vi "2D scan.vi"(5 "FIB Para":T4={"Z-step (nm)"=5.0, "Emission max"=4.0, "Emission min"=1.6, "Milling current (nA)"=1.2, "Enable alarm"=TRUE} {"Milling current (nA)" format="%.1g"}, 6 "Options":T6={"GetInfo"=TRUE, "Set Det A para"=TRUE, "Set WD"=FALSE, "Set Mag"=TRUE, "Set stig"=FALSE, "Display"=TRUE, "Save"=TRUE, "Detector A"=TRUE, "Detector B"=TRUE, "Detector C"=FALSE, "Detector D"=FALSE, "Inverse A"=FALSE, "Inverse B"=FALSE, "Inverse C"=FALSE, "Inverse D"=FALSE, "Inverse PNG"=FALSE, "Freeze"=TRUE, "PNG only"=TRUE}, 7 "File Info":cluster{"File path":path, "Notes":string}={"File path"=path "T:/Images", "Notes"=""}, 8 "Scan Para":T7={"X resolution"=1024, "Y resolution"=1024, "X center"=0.0, "Y center"=0.0, "X size (V)"=20.0, "Y size (V)"=20.0, "X stig"=0.0, "Y stig"=0.0, "Scan rate (Hz)"=1000000, "Oversampling"=4, "Read AI delay (samples)"=1, "Frame line rampdown ratio"=0.1, "Pixel size (nm)"=5.0, "WD"=4.0} {"WD" format="%#_7g"; "Frame line rampdown ratio" min=-1.0 max=1.0 step=0.05 format="%.2g"; "Scan rate (Hz)" max=4000000 format="%.2e"}, 9 "Det Info":T8={"Brightness A"=40.0, "Contrast A"=26.0, "Detector B name"="ESB @ 1.0 kV", "Brightness B"=40.0, "Contrast B"=40.0, "Detector C name"="PMT @ 6.0", "Detector D name"="Detector D"}, 10 "HW Config":T9={"SEM X coil"="PXI1Slot7/ao0", "SEM Y coil"="PXI1Slot7/ao1", "Detector A"="PXI1Slot7/ai0", "Detector B"="PXI1Slot7/ai1", "Detector C"="PXI1Slot7/ai2", "Detector D"="PXI1Slot7/ai3", "Det min (V)"=-10.0, "Det max (V)"=10.0, "COM port"="COM1", "Detector FIB-NI auto switch"="PXI1Slot7/port0/line0", "Machine Type"=0} {"Machine Type" items=["Feiss", "NVision"]}) -> (0 "Image Focus Index":T1, 1 "FIB parameters":T3, 2 "SEM parameters":T2={"Detector A"="", "Detector B"="Detecter B name", "Brightness A"=0.0, "Contrast A"=0.0, "Brightness B"=0.0, "Contrast B"=0.0, "Magnification"=0.0, "Pixel size"=0.0, "Working distance"=0.0, "EHT"=0.0, "Aperture"=0, "High current mode"=0, "Probe current"=0.0, "Scan rotation"=0.0, "Chamber vac"=0.0, "Gun vac"=0.0, "Beam shift X"=0.0, "Beam shift Y"=0.0, "Stig X"=0.0, "Stig Y"=0.0, "Alignment X"=0.0, "Alignment Y"=0.0, "Stage X"=0.0, "Stage Y"=0.0, "Stage Z"=0.0, "Stage T"=0.0, "Stage R"=0.0, "Stage M"=0.0}, 3 "Info & Status":T5={"AO SampClk.MaxRate"=2500000.0, "AI SampClk.MaxRate"=4000000.0, "AO rate"=1000000.0, "Scan speed"=4, "Detector number"=2, "X min (V)"=-10.0, "X max (V)"=10.0, "X min index"=0, "X max index"=1024, "AO multiline"=512, "Decimating factor"=2, "AvailSampPerChan"=17560, "AO scan line"=1024, "Total pixels recorded"=1048576, "Total lines scanned"=1024, "Scan time (m)"=0.0, "Scan time (s)"=1.153024, "Remaining time (m)"=0, "Remaining time (s)"=0} {"AvailSampPerChan" scale=0.0..1000000.0; "Scan time (s)" format="%.3f"; "Total pixels recorded" scale=0.0..1048576.0; "Scan speed" scale=1.0..15.0; "AO rate" format="%#_3e"})   [LabVIEW 2012]
uses:
  <vilib>/Utility/error.llb/DialogType.ctl
  <vilib>/DAQmx/write.llb/DAQmx Write (Digital Bool 1Line 1Point).vi
  <vilib>/DAQmx/read.llb/DAQmx Read (Raw 1D I16).vi
  <vilib>/DAQmx/write.llb/DAQmx Write (Analog 2D DBL NChan NSamp).vi
  <vilib>/DAQmx/create/channels.llb/DAQmx Create Channel (AI-Voltage-Basic).vi
  <vilib>/DAQmx/create/channels.llb/DAQmx Create Channel (AO-Voltage-Basic).vi
  <vilib>/DAQmx/create/channels.llb/DAQmx Create Channel (DO-Digital Output).vi
  <vilib>/DAQmx/miscellaneous.llb/DAQmx Fill In Error Info.vi
  <vilib>/DAQmx/configure/timing.llb/DAQmx Timing (Sample Clock).vi
  <vilib>/DAQmx/configure/trigger.llb/DAQmx Start Trigger (Digital Edge).vi
  <vilib>/Analysis/2dsp.llb/Decimate (single shot, DBL).vi
  <resource>/objmgr/daqmx.rc
  <vilib>/Analysis/NI_AALPro.lvlib
panel:
  out "PNG only":bool
  out "Eval D":i16[][](graph)
  out "Eval C":i16[][](graph)
  out "Eval B":i16[][](graph)
  out "Eval A":i16[][](graph)
  out "Freeze":bool
  out "Detector FIB-NI auto switch":tag
  out "GetInfo":bool
  out "Set X stig":bool=TRUE
  out "Y stig":dbl
  out "X stig":dbl
  out "Total time":dbl=1.153024
  in  "stop":bool=TRUE
  out "Det max (V)":dbl=10.0
  out "Det min (V)":dbl=-10.0
  out "Y max set":dbl=10.0
  out "Y min set":dbl=-10.0
  out "X max set":dbl=10.0
  out "X min set":dbl=-10.0
  in  "AvailSampPerChan":u32(slide)=17560 scale=0.0..1000000.0
  in  "AO scan line":u32=1024
  in  "AO multiline":u32=512
  in  "Decimating factor":u16=2
  in  "Remaining time (m)":u16
  in  "Remaining time (s)":u8
  in  "Scan time (s)":dbl=1.153024 format="%.3f"
  in  "Scan time (m)":dbl
  in  "Total lines scanned":i32=1024
  in  "Total pixels recorded":i32(slide)=1048576 scale=-1.0..1048576.0
  in  "X max (V)":dbl=10.0
  in  "X min (V)":dbl=-10.0
  in  "X min index":i32
  in  "X max index":i32=1024
  in  "Scan speed":u8(slide)=4 scale=1.0..15.0
  in  "AO rate":dbl=1000000.0 caption="Scanning rate" format="%#_3e"
  in  "Detector number":u8=2
  in  "AI SampClk.MaxRate":dbl=4000000.0
  in  "AO SampClk.MaxRate":dbl=2500000.0
  out "Det A Img":i16[][](graph)
  out "Det B Img":i16[][](graph)
  out "Det C Img":i16[][](graph)
  out "Det D Img":i16[][](graph)
  out "Notes":string
  out "File path":path=path "T:/Images/SW Tests"
  out "Inverse PNG":bool=TRUE
  out "Inverse D":bool
  out "Inverse C":bool
  out "Inverse B":bool
  out "Inverse A":bool
  out "Detector D":bool
  out "Detector C":bool
  out "Detector B":bool=TRUE
  out "Detector A":bool=TRUE
  out "Save":bool=TRUE
  out "Display":bool
  out "Set Mag":bool=TRUE
  out "Set WD":bool
  out "Set Det A para":bool=TRUE
  out "Z-step (nm)":dbl
  out "WD":dbl=6.0
  out "Pixel size (nm)":dbl=100.0
  out "Frame line rampdown ratio":dbl=0.1
  out "Read AI delay (samples)":i16=1
  out "Oversampling":u16=4
  out "Scan rate (Hz)":u32=1000000
  out "Y size (V)":dbl=20.0
  out "X size (V)":dbl=20.0
  out "Y center":dbl
  out "X center":dbl
  out "Y resolution":u32=1024
  out "X resolution":u32=1024
  out "Detector D name":string="Detector D"
  out "Detector C name":string="PMT @ 6.0"
  out "Contrast B":dbl=40.0
  out "Brightness B":dbl=40.0
  out "Detector B name":string="ESB @ 1.0 kV"
  out "Contrast A":dbl=26.0
  out "Brightness A":dbl=40.0
  out "COM port":refnum<visa-resource-name>="COM1"
  out "Det D I/O":tag="PXI1Slot3/ai3"
  out "Det C I/O":tag="PXI1Slot3/ai2"
  out "Det B I/O":tag="PXI1Slot3/ai1"
  out "Det A I/O":tag="PXI1Slot3/ai0"
  out "SEM Y coil":tag="PXI1Slot3/ao1"
  out "SEM X coil":tag="PXI1Slot3/ao0"
  out "File name":path=path "T:/Images/SW Tests/Y2010/M03/D26/Neon_10-03-26_153931.dat"
  out "Header done?":bool=TRUE
  # "Hardware Configuration"
  # "FIBBing Parameters"
  # "Detectors Information"
  # "Scanning Parameters"
  # "Emssion Alarm (uA)"
  # "Hz"
  # "Scanning time"
  # "m"
  # "s"
  # "Remaining time"
  # "m"
  # "s"
  # "Det"
  # "Detector A"
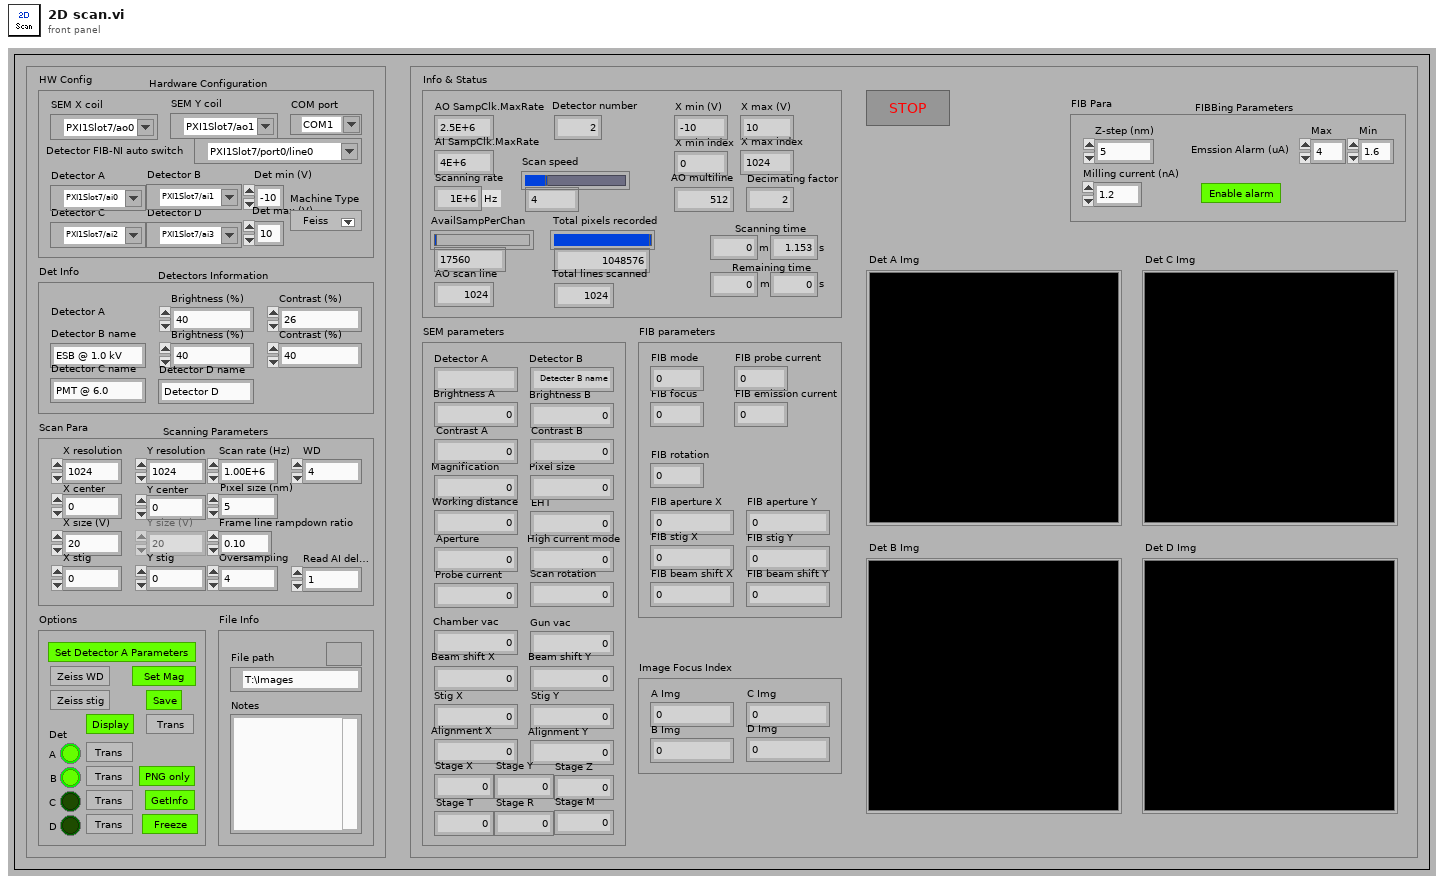
[diagram p1: front panel]
types:
  T1 = cluster{"A Img Focus Index":dbl, "B Img Focus Index":dbl, "C Img Focus Index":dbl, "D Img Focus Index":dbl}
  T2 = cluster{"Detector A":string, "Detector B":string, "Brightness A":sgl, "Contrast A":sgl, "Brightness B":sgl, "Contrast B":sgl, "Magnification":sgl, "Pixel size":sgl, "Working distance":sgl, "EHT":sgl, "Aperture":u8, "High current mode":u8, "Probe current":sgl, "Scan rotation":sgl, "Chamber vac":sgl, "Gun vac":sgl, "Beam shift X":sgl, "Beam shift Y":sgl, "Stig X":sgl, "Stig Y":sgl, "Alignment X":sgl, "Alignment Y":sgl, "Stage X":sgl, "Stage Y":sgl, "Stage Z":sgl, "Stage T":sgl, "Stage R":sgl, "Stage M":sgl}
  T3 = cluster{"FIB mode":u8, "FIB focus":sgl, "FIB probe current":u8, "FIB emission current":sgl, "FIB rotation":sgl, "FIB aperture X":sgl, "FIB aperture Y":sgl, "FIB stig X":sgl, "FIB stig Y":sgl, "FIB beam shift X":sgl, "FIB beam shift Y":sgl}
  T4 = cluster{"Z-step (nm)":dbl, "Emission max":dbl, "Emission min":dbl, "Milling current (nA)":sgl, "Enable alarm":bool}
  T5 = cluster{"AO SampClk.MaxRate":dbl, "AI SampClk.MaxRate":dbl, "AO rate":dbl, "Scan speed":u8, "Detector number":u8, "X min (V)":dbl, "X max (V)":dbl, "X min index":i32, "X max index":i32, "AO multiline":u32, "Decimating factor":u16, "AvailSampPerChan":u32, "AO scan line":u32, "Total pixels recorded":i32, "Total lines scanned":i32, "Scan time (m)":dbl, "Scan time (s)":dbl, "Remaining time (m)":u16, "Remaining time (s)":u8}
  T6 = cluster{"GetInfo":bool, "Set Det A para":bool, "Set WD":bool, "Set Mag":bool, "Set stig":bool, "Display":bool, "Save":bool, "Detector A":bool, "Detector B":bool, "Detector C":bool, "Detector D":bool, "Inverse A":bool, "Inverse B":bool, "Inverse C":bool, "Inverse D":bool, "Inverse PNG":bool, "Freeze":bool, "PNG only":bool}
  T7 = cluster{"X resolution":u32, "Y resolution":u32, "X center":dbl, "Y center":dbl, "X size (V)":dbl, "Y size (V)":dbl, "X stig":dbl, "Y stig":dbl, "Scan rate (Hz)":u32, "Oversampling":u16, "Read AI delay (samples)":i16, "Frame line rampdown ratio":dbl, "Pixel size (nm)":dbl, "WD":dbl}
  T8 = cluster{"Brightness A":dbl, "Contrast A":dbl, "Detector B name":string, "Brightness B":dbl, "Contrast B":dbl, "Detector C name":string, "Detector D name":string}
  T9 = cluster{"SEM X coil":tag, "SEM Y coil":tag, "Detector A":tag, "Detector B":tag, "Detector C":tag, "Detector D":tag, "Det min (V)":dbl, "Det max (V)":dbl, "COM port":refnum<visa-resource-name>, "Detector FIB-NI auto switch":tag, "Machine Type":u8}
  T10 = enum16{"SEM", "FIB", "Milling", "SEM + FIB", "Mill + SEM", "SEM Drift Correction", "FIB Drift Correction", "No Beam", "External", "External + SEM"}
  T11 = enum16{"open", "replace", "create", "open or create", "replace or create", "replace or create with confirmation"}
  T12 = typedef "DialogType.ctl" = u16
  T13 = cluster{"X resolution":u32, "Y resolution":u32, "Oversampling":u16, "Read AI delay (samples)":i16, "Scan speed":u8, "AO rate":dbl, "Frame line rampdown ratio":dbl, "X min (V)":dbl, "X max (V)":dbl}
  T14 = cluster{"Detector A":bool, "Detector B":bool, "Detector C":bool, "Detector D":bool}
  T15 = cluster{"Detector C name":string, "Detector D name":string}
  T16 = typedef "imagedata.ctl" = cluster{"image type":i32, "image depth":i32, "image":u8[], "mask":u8[], "colors":u32[], "Rectangle":cluster{"left":i16, "top":i16, "right":i16, "bottom":i16}}
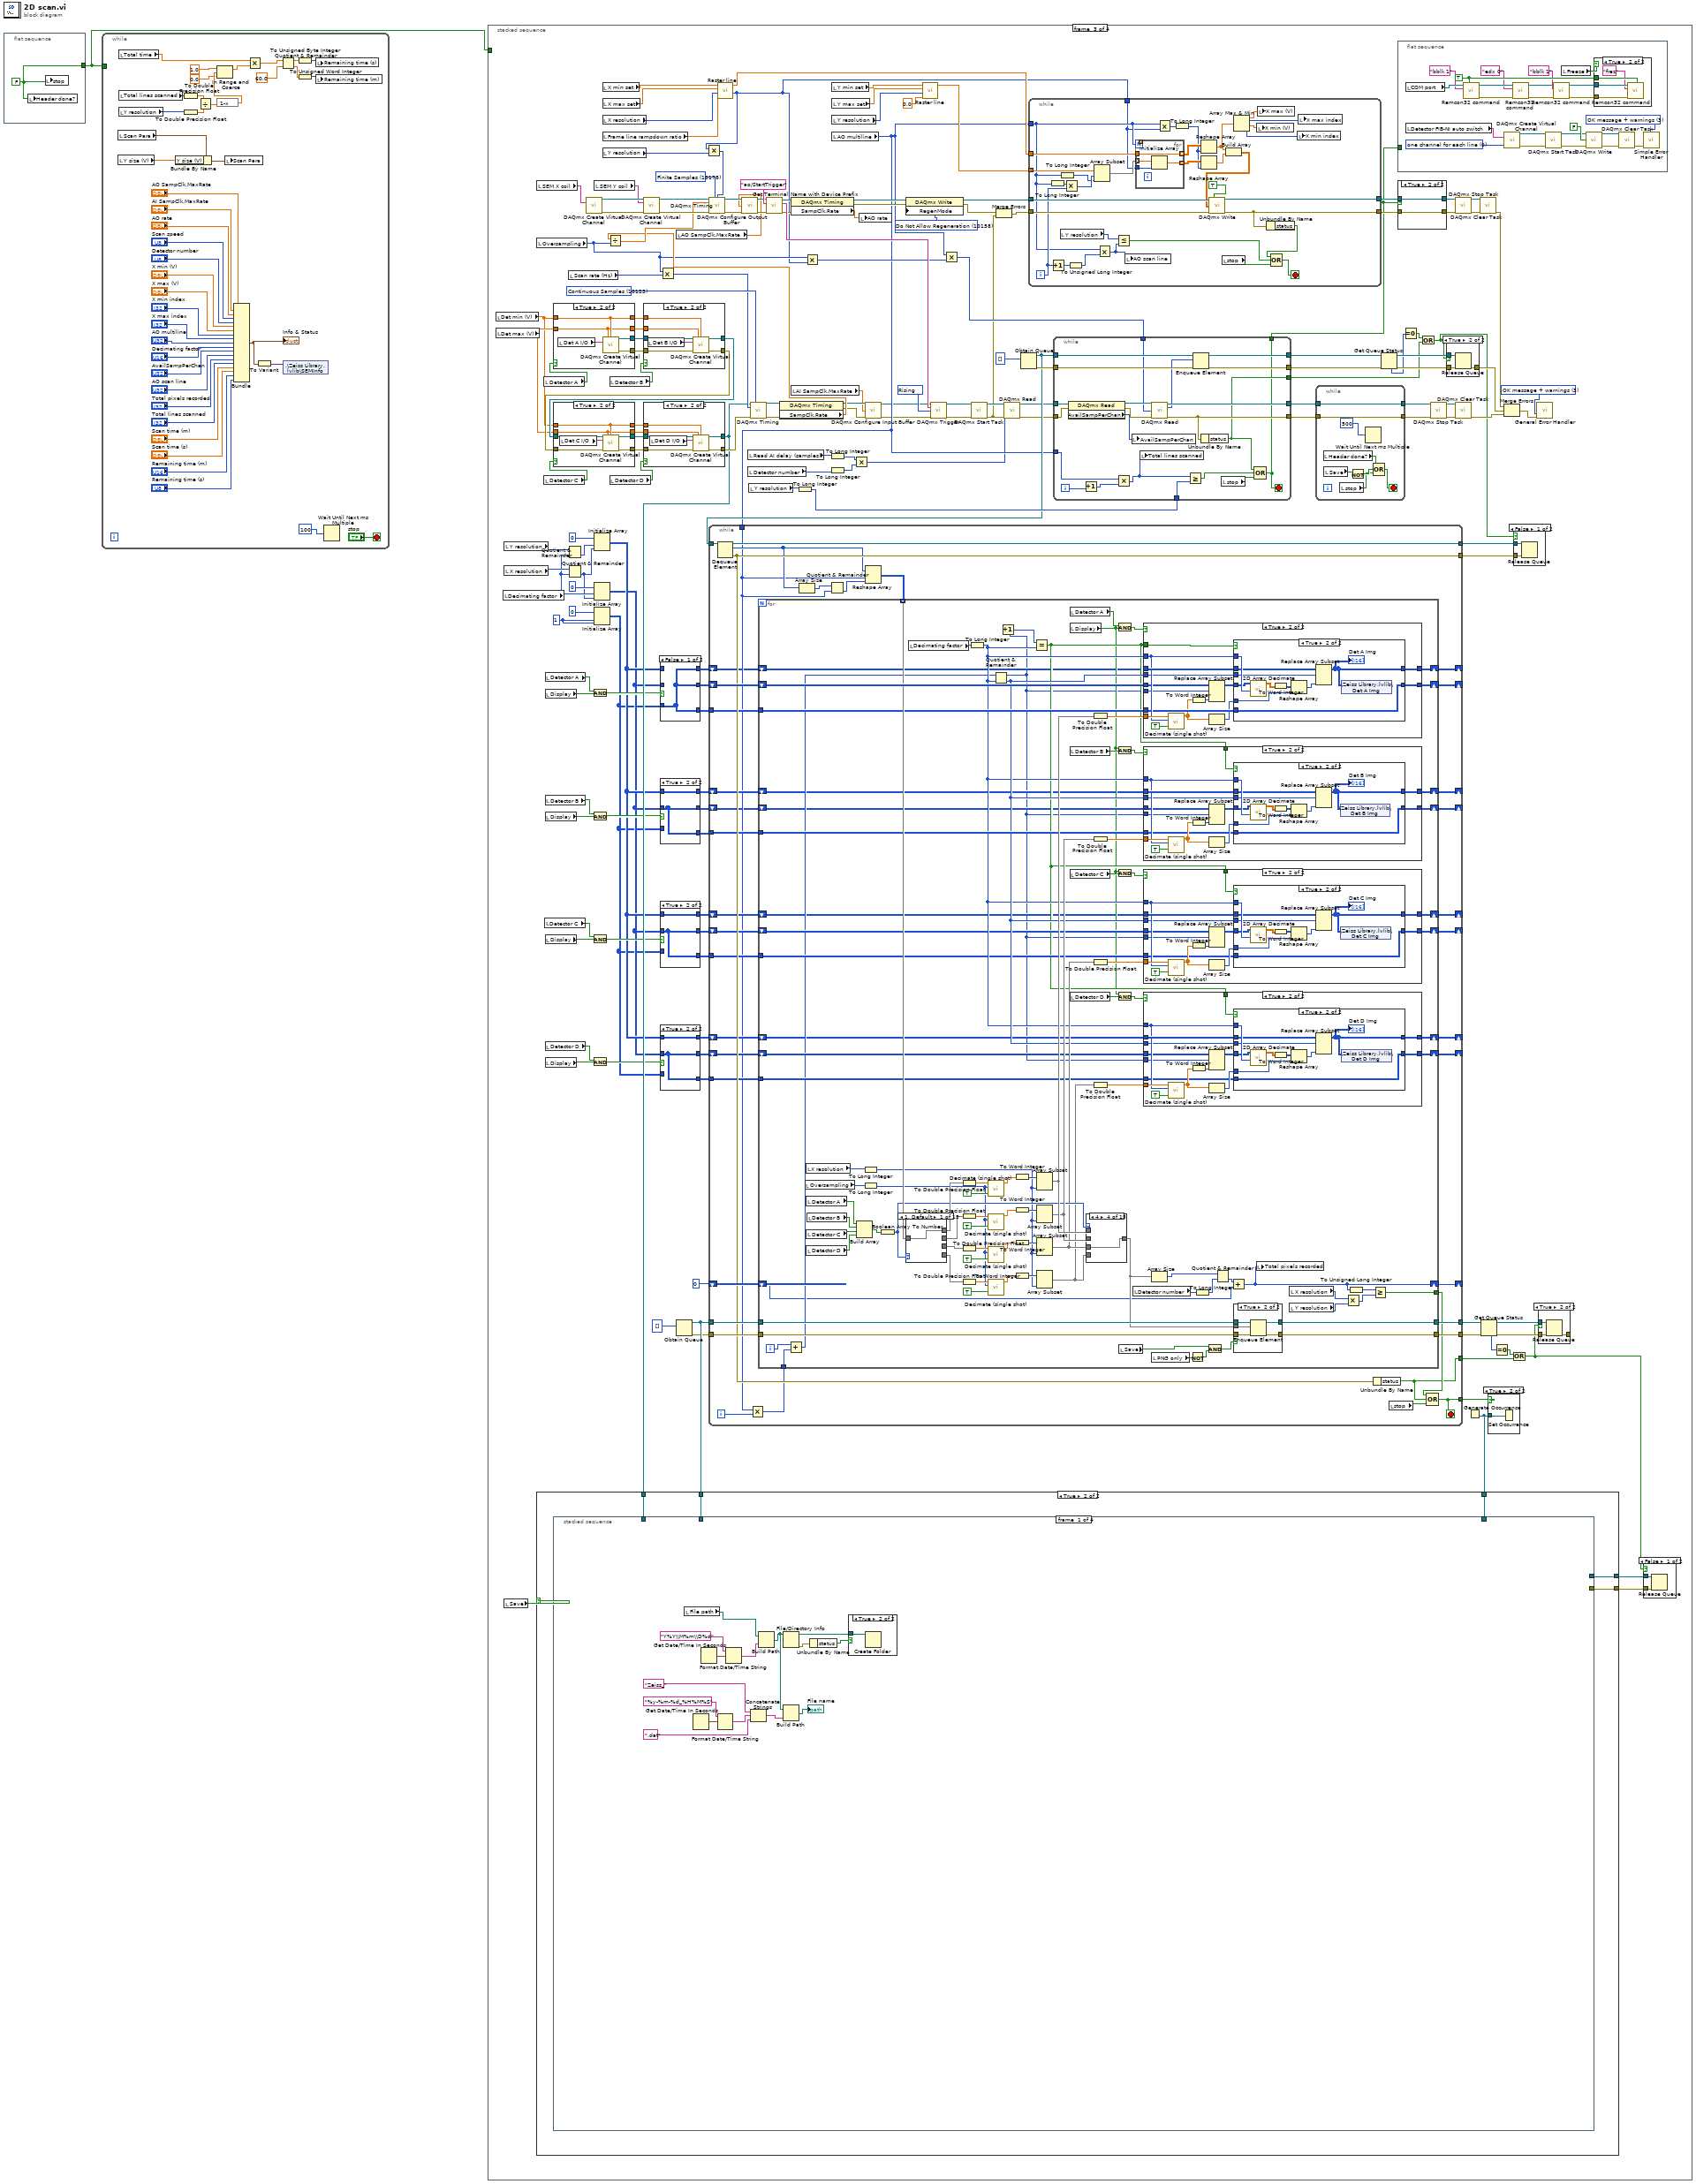
[diagram p0: block diagram]
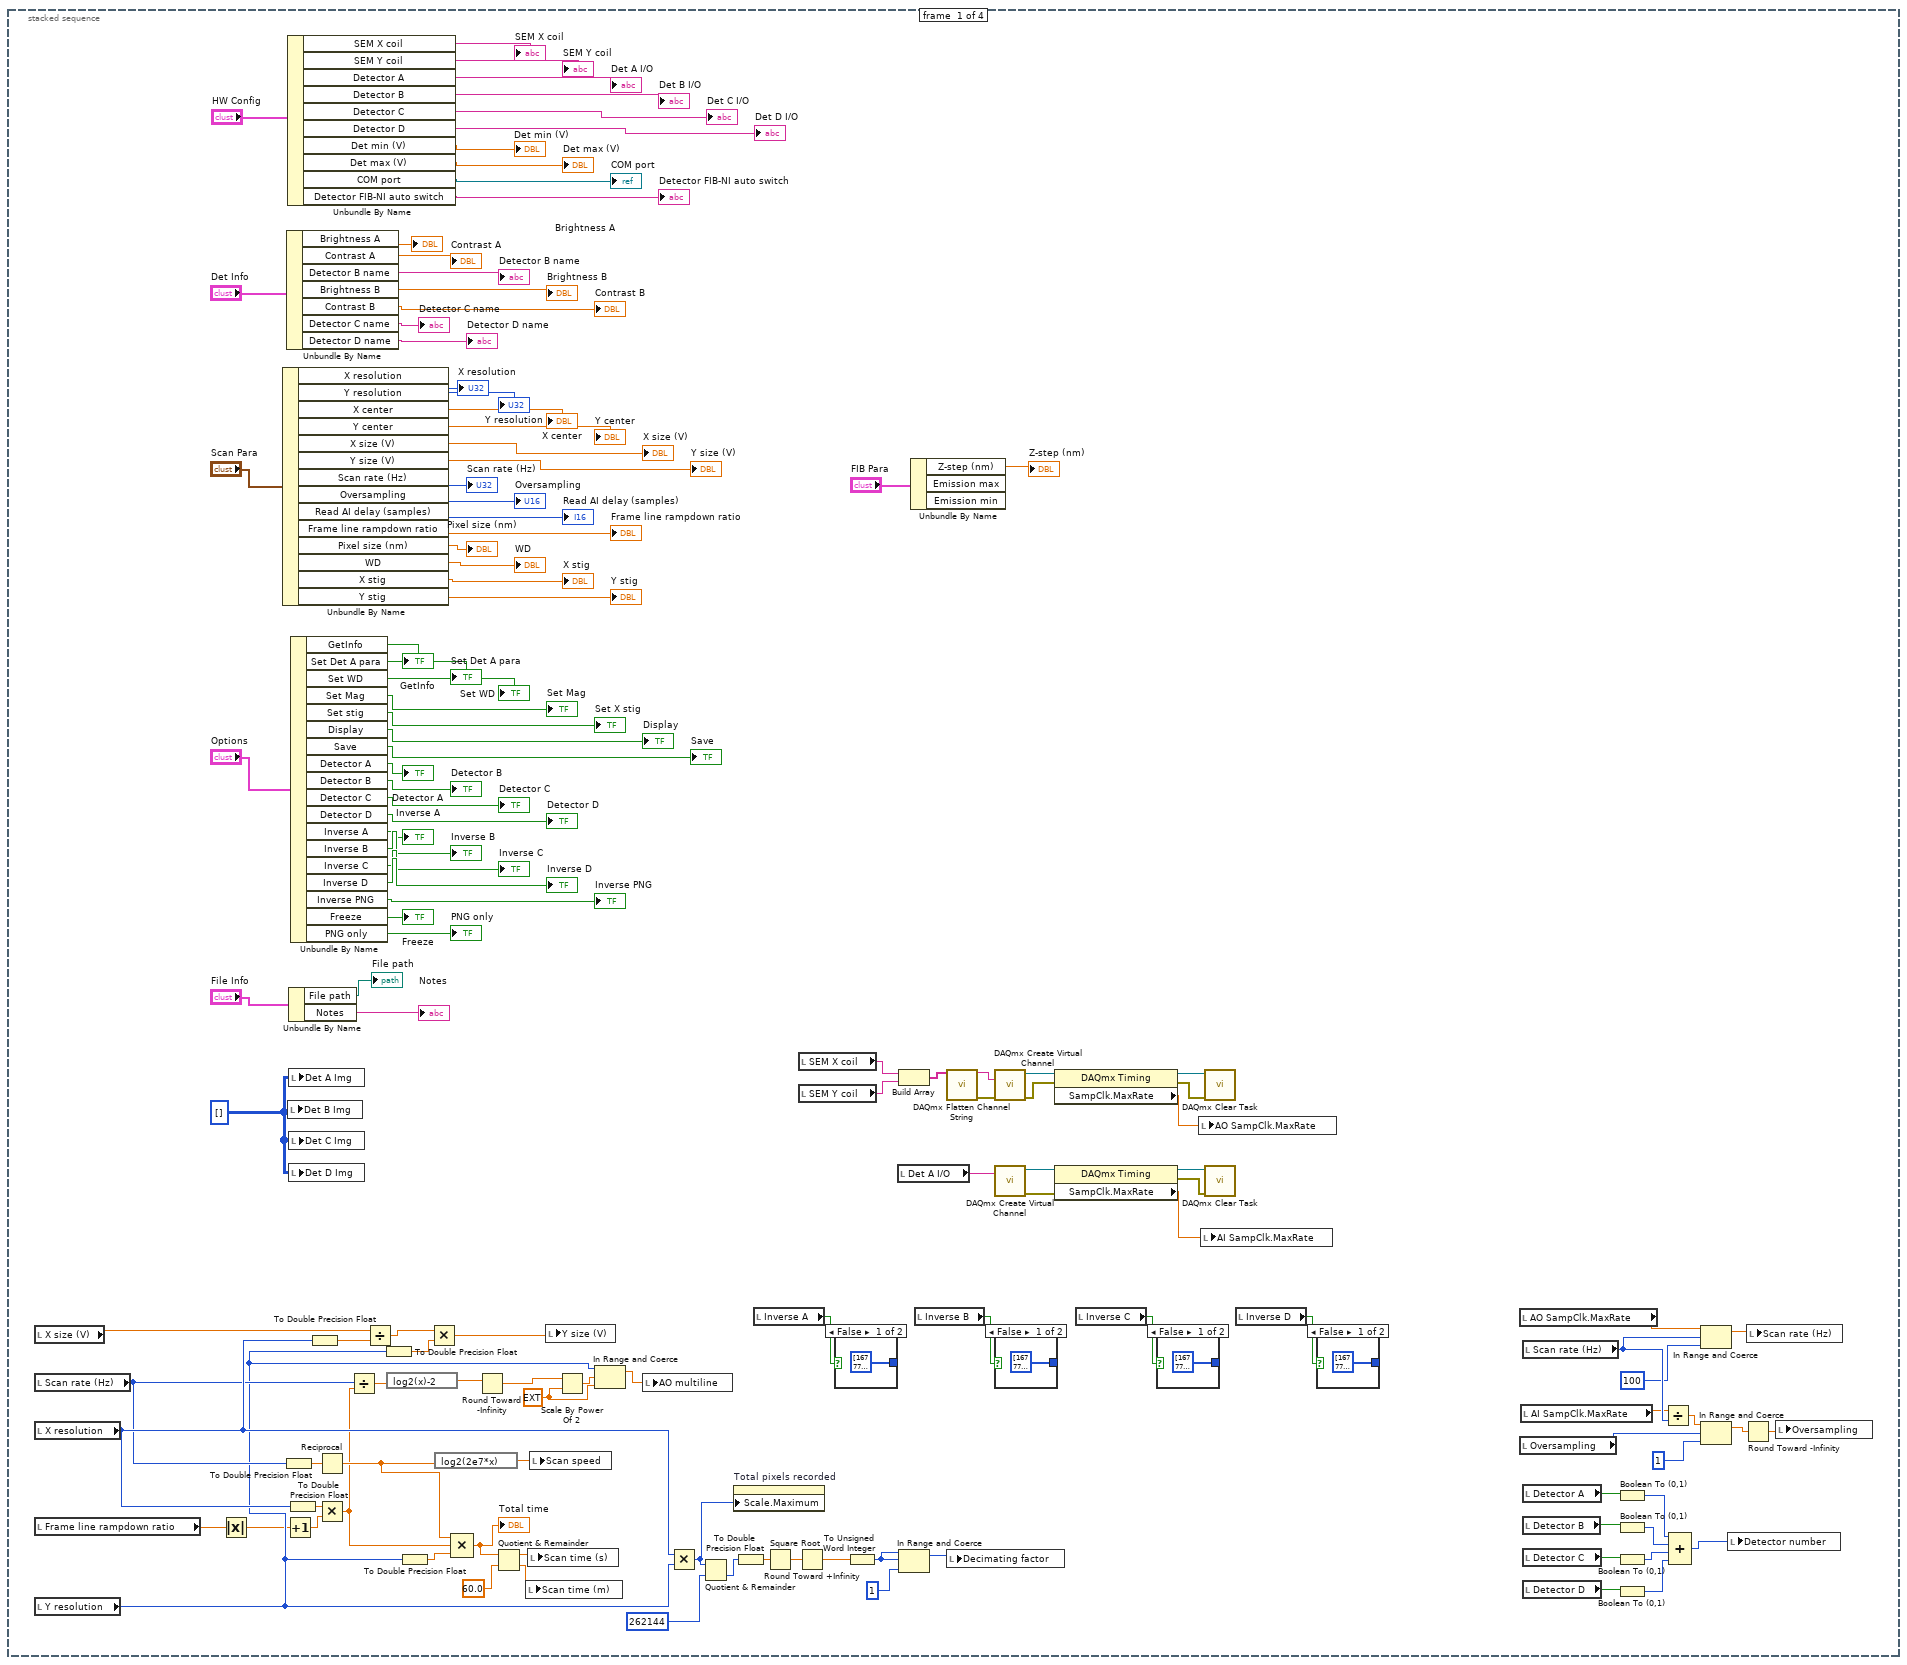
[diagram p2: hidden frame]
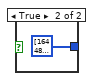
[diagram p3: hidden frame]
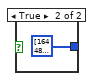
[diagram p4: hidden frame]
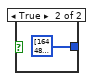
[diagram p5: hidden frame]
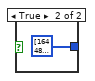
[diagram p6: hidden frame]
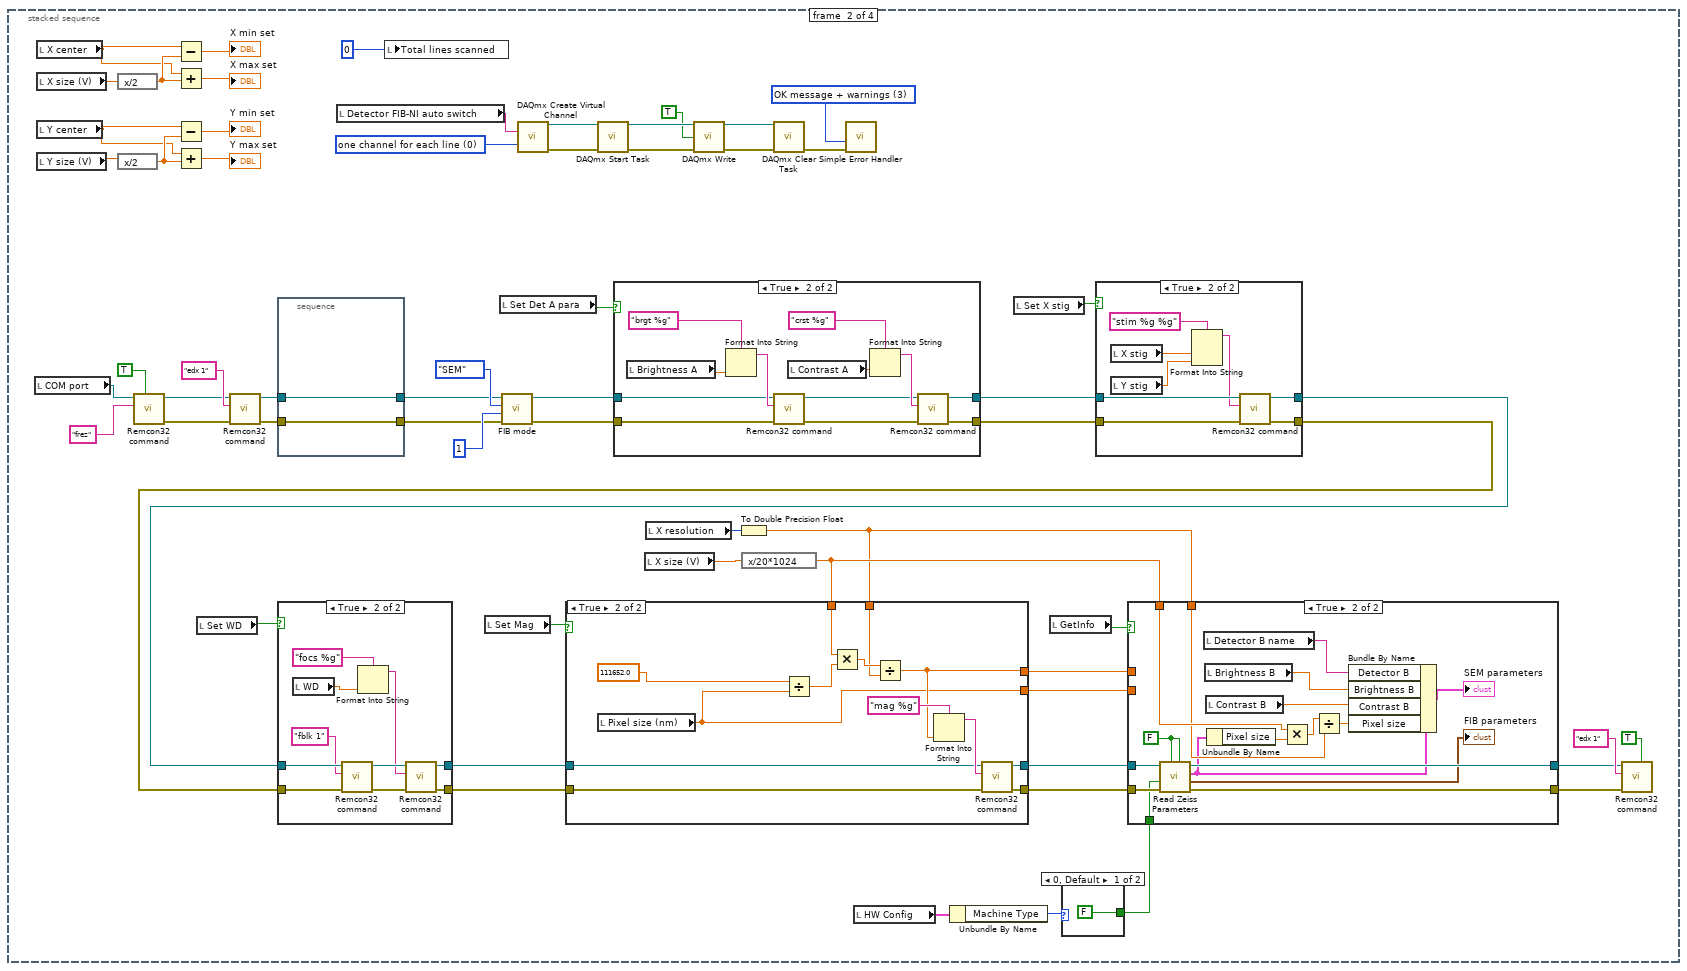
[diagram p7: hidden frame]
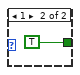
[diagram p8: hidden frame]
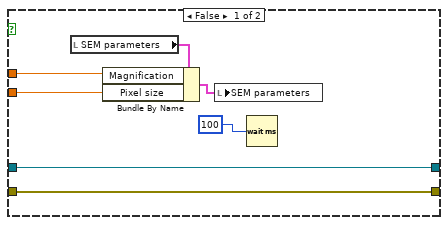
[diagram p9: hidden frame]
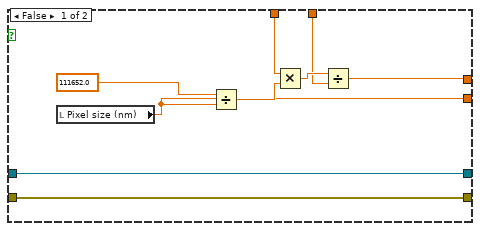
[diagram p12: hidden frame]
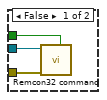
[diagram p14: hidden frame]
diagram:
  n1 = flat-sequence {
    tunnel: [w2] -> w1
    frame #0 {
      w2 = FALSE ("stop")
      n2 = local write "Header done?"(w2) -> ()
      n3 = local write "stop"(w2) -> ()
    }
  }
  n4 = while {
    tunnel: w1 -> [_]
    stop <- "stop" stop-if-true
    n5 = local read "Scan Para"() -> (w24:T7)
    n6 = local read "Y size (V)"() -> (w22:dbl)
    n7 = local read "Total time"() -> (w21:dbl)
    n8 = local read "Total lines scanned"() -> (w20:i32)
    n9 = local read "Y resolution"() -> (w9:u32)
    n10 = Bundle By Name(cluster=w24, "Y size (V)"=w22) -> (w23:T7)
    n11 = To Double Precision Float(number=w20) -> (double precision float=w13:dbl)
    n12 = To Double Precision Float(number=w9) -> (double precision float=w14:dbl)
    n13 = Divide(x=w13, y=w14) -> (x/y=w19:dbl)
    n14 = expression code="1-x"(w19) -> (w6:dbl)
    n15 = In Range and Coerce(upper limit=1.0, x=w6, lower limit=0.0) -> (coerced(x)=w3:dbl)  [unwired: 1 out]
    n16 = local write "Scan Para"(w23) -> ()
    n17 = Bundle("AO SampClk.MaxRate"="AO SampClk.MaxRate", "AI SampClk.MaxRate"="AI SampClk.MaxRate", "AO rate"="AO rate", "Scan speed"="Scan speed", "Detector number"="Detector number", "X min (V)"="X min (V)", "X max (V)"="X max (V)", "X min index"="X min index", "X max index"="X max index", "AO multiline"="AO multiline", "Decimating factor"="Decimating factor", "AvailSampPerChan"="AvailSampPerChan", "AO scan line"="AO scan line", "Total pixels recorded"="Total pixels recorded", "Total lines scanned"="Total lines scanned", "Scan time (m)"="Scan time (m)", "Scan time (s)"="Scan time (s)", "Remaining time (m)"="Remaining time (m)", "Remaining time (s)"="Remaining time (s)") -> (w7:T5)  [unwired: 1 out]
    "Info & Status" <- w7
    n18 = Multiply(x=w21, y=w3) -> (x*y=w15:dbl)
    n19 = To Variant(anything=w7) -> (Variant=w8:variant)
    n20 = Quotient & Remainder(x=w15, y=60.0) -> (x-y*floor(x/y)=w18:dbl, floor(x/y)=w17:dbl)
    n21 = shared-variable ".\\Zeiss Library.lvlib\\SEMInfo"(w8) -> ()  [unwired: 2 out]
    n22 = To Unsigned Byte Integer(number=w18) -> (unsigned 8bit integer=w11:u8)
    n23 = To Unsigned Word Integer(number=w17) -> (unsigned 16bit integer=w12:u16)
    n24 = local write "Remaining time (s)"(w11) -> ()
    n25 = local write "Remaining time (m)"(w12) -> ()
    n26 = Wait Until Next ms Multiple(millisecond multiple=u32 100) -> ()  [unwired: 1 out]
  }
  n27 = stacked-sequence {
    tunnel: w1 -> [_ _ _ _]
    frame #0 {
      w112 = i16[][] [] ("SEM")
      w164 = ext 1.0 ("x")
      n28 = local read "X size (V)"() -> (w167:dbl)
      n29 = local read "Scan rate (Hz)"() -> (w169:u32)
      n30 = local read "X resolution"() -> (w170:u32)
      n31 = local read "Frame line rampdown ratio"() -> (w171:dbl)
      n32 = local read "Y resolution"() -> (w168:u32)
      n33 = Absolute Value(x=w171) -> (abs(x)=w51:dbl)
      n34 = Unbundle By Name("Scan Para") -> ("X resolution"=→"X resolution":u32, "Y resolution"=→"Y resolution":u32, "X center"=→"X center":dbl, "Y center"=→"Y center":dbl, "X size (V)"=→"X size (V)":dbl, "Y size (V)"=→"Y size (V)":dbl, "Scan rate (Hz)"=→"Scan rate (Hz)":u32, "Oversampling"=→"Oversampling":u16, "Read AI delay (samples)"=→"Read AI delay (samples)":i16, "Frame line rampdown ratio"=→"Frame line rampdown ratio":dbl, "Pixel size (nm)"=→"Pixel size (nm)":dbl, "WD"=→"WD":dbl, "X stig"=→"X stig":dbl, "Y stig"=→"Y stig":dbl)
      n35 = To Double Precision Float(number=w169) -> (double precision float=w154:dbl)
      n36 = Increment(x=w51) -> (x+1=w149:dbl)
      n37 = Unbundle By Name("Det Info") -> ("Brightness A"=→"Brightness A":dbl, "Contrast A"=→"Contrast A":dbl, "Detector B name"=→"Detector B name":string, "Brightness B"=→"Brightness B":dbl, "Contrast B"=→"Contrast B":dbl, "Detector C name"=→"Detector C name":string, "Detector D name"=→"Detector D name":string)
      n38 = Unbundle By Name("HW Config") -> ("SEM X coil"=→"SEM X coil":tag, "SEM Y coil"=→"SEM Y coil":tag, "Detector A"=→"Det A I/O":tag, "Detector B"=→"Det B I/O":tag, "Detector C"=→"Det C I/O":tag, "Detector D"=→"Det D I/O":tag, "Det min (V)"=→"Det min (V)":dbl, "Det max (V)"=→"Det max (V)":dbl, "COM port"=→"COM port":refnum<visa-resource-name>, "Detector FIB-NI auto switch"=→"Detector FIB-NI auto switch":tag)
      n39 = local write "Det B Img"(w112) -> ()
      n40 = To Double Precision Float(number=w170) -> (double precision float=w155:dbl)
      n41 = Unbundle By Name("File Info") -> ("File path"=→"File path":path, "Notes"=→"Notes":string)
      n42 = local write "Det A Img"(w112) -> ()
      n43 = local write "Det C Img"(w112) -> ()
      n44 = local write "Det D Img"(w112) -> ()
      n45 = Unbundle By Name("Options") -> ("GetInfo"=→"GetInfo":bool, "Set Det A para"=→"Set Det A para":bool, "Set WD"=→"Set WD":bool, "Set Mag"=→"Set Mag":bool, "Set stig"=→"Set X stig":bool, "Display"=→"Display":bool, "Save"=→"Save":bool, "Detector A"=→"Detector A":bool, "Detector B"=→"Detector B":bool, "Detector C"=→"Detector C":bool, "Detector D"=→"Detector D":bool, "Inverse A"=→"Inverse A":bool, "Inverse B"=→"Inverse B":bool, "Inverse C"=→"Inverse C":bool, "Inverse D"=→"Inverse D":bool, "Inverse PNG"=→"Inverse PNG":bool, "Freeze"=→"Freeze":bool, "PNG only"=→"PNG only":bool)
      n46 = To Double Precision Float(number=w170) -> (double precision float=w153:dbl)
      n47 = Reciprocal(x=w154) -> (1/x=w150:dbl)
      n48 = Multiply(x=w155, y=w149) -> (x*y=w49:dbl)
      n49 = Divide(x=w169, y=w49) -> (x/y=w161:dbl)
      n50 = Divide(x=w167, y=w153) -> (x/y=w152:dbl)
      n51 = To Double Precision Float(number=w168) -> (double precision float=w156:dbl)
      n52 = expression code="log2(x)-2"(w161) -> (w162:dbl)
      n53 = To Double Precision Float(number=w168) -> (double precision float=w157:dbl)
      n54 = Multiply(x=w152, y=w156) -> (x*y=w166:dbl)
      n55 = expression code="log2(2e7*x)"(w150) -> (w172:dbl)
      n56 = Compound Arithmetic op=MULTIPLY(w150, w49, w157) -> (w151:dbl)
      "Total time" <- w151
      n57 = Round Toward -Infinity(1:w162) -> (0:w165:dbl)
      n58 = Quotient & Remainder(x=w151, y=60.0) -> (x-y*floor(x/y)=w174:dbl, floor(x/y)=w173:dbl)
      n59 = local write "Scan time (m)"(w173) -> ()
      n60 = local write "Scan time (s)"(w174) -> ()
      n61 = local write "Scan speed"(w172) -> ()
      n62 = local write "Y size (V)"(w166) -> ()
      n63 = Scale By Power Of 2(n=w165, x=w164) -> (x*2^n=w163:ext)
      n64 = In Range and Coerce(upper limit=w168, x=w163, lower limit=w164) -> (coerced(x)=w50:ext)  [unwired: 1 out]
      n65 = local write "AO multiline"(w50) -> ()
      n66 = Multiply(x=w170, y=w168) -> (x*y=w148:u32)
      n67 = Quotient & Remainder(x=w148, y=u32 262144) -> (floor(x/y)=w146:u32)  [unwired: 1 out]
      n68 = property on="Total pixels recorded" class="Slide (strict)"("Scale.Maximum"=w148) -> ()  [unwired: 2 in, 2 out]
      n69 = To Double Precision Float(number=w146) -> (double precision float=w159:dbl)
      n70 = local read "Inverse A"() -> (w175:bool)
      n71 = Square Root(x=w159) -> (sqrt(x)=w147:dbl)
      n72 = Round Toward +Infinity(x=w147) -> (ceil(x): smallest int >= x=w160:dbl)
      n73 = local read "SEM X coil"() -> (w115:tag)
      n74 = local read "SEM Y coil"() -> (w114:tag)
      n75 = case shown="False" w175 {
        tunnel: [u32[] [16777222, 65793, 131586, 197379, 263172, 328965, 394758, 460551, 526344, 592137, 657930, 723723, 789516, 855309, 921102, 986895, 1052688, 1118481, 1184274, 1250067, 1315860, 1381653, 1447446, 1513239, 1579032, 1644825, 1710618, 1776411, 1842204, 1907997, 1973790, 2039583, 2105376, 2171169, 2236962, 2302755, 2368548, 2434341, 2500134, 2565927, 2631720, 2697513, 2763306, 2829099, 2894892, 2960685, 3026478, 3092271, 3158064, 3223857, 3289650, 3355443, 3421236, 3487029, 3552822, 3618615, 3684408, 3750201, 3815994, 3881787, 3947580, 4013373, 4079166, 4144959, 4210752, 4276545, 4342338, 4408131, 4473924, 4539717, 4605510, 4671303, 4737096, 4802889, 4868682, 4934475, 5000268, 5066061, 5131854, 5197647, 5263440, 5329233, 5395026, 5460819, 5526612, 5592405, 5658198, 5723991, 5789784, 5855577, 5921370, 5987163, 6052956, 6118749, 6184542, 6250335, 6316128, 6381921, 6447714, 6513507, 6579300, 6645093, 6710886, 6776679, 6842472, 6908265, 6974058, 7039851, 7105644, 7171437, 7237230, 7303023, 7368816, 7434609, 7500402, 7566195, 7631988, 7697781, 7763574, 7829367, 7895160, 7960953, 8026746, 8092539, 8158332, 8224125, 8289918, 8355711, 8421504, 8487297, 8553090, 8618883, 8684676, 8750469, 8816262, 8882055, 8947848, 9013641, 9079434, 9145227, 9211020, 9276813, 9342606, 9408399, 9474192, 9539985, 9605778, 9671571, 9737364, 9803157, 9868950, 9934743, 10000536, 10066329, 10132122, 10197915, 10263708, 10329501, 10395294, 10461087, 10526880, 10592673, 10658466, 10724259, 10790052, 10855845, 10921638, 10987431, 11053224, 11119017, 11184810, 11250603, 11316396, 11382189, 11447982, 11513775, 11579568, 11645361, 11711154, 11776947, 11842740, 11908533, 11974326, 12040119, 12105912, 12171705, 12237498, 12303291, 12369084, 12434877, 12500670, 12566463, 12632256, 12698049, 12763842, 12829635, 12895428, 12961221, 13027014, 13092807, 13158600, 13224393, 13290186, 13355979, 13421772, 13487565, 13553358, 13619151, 13684944, 13750737, 13816530, 13882323, 13948116, 14013909, 14079702, 14145495, 14211288, 14277081, 14342874, 14408667, 14474460, 14540253, 14606046, 14671839, 14737632, 14803425, 14869218, 14935011, 15000804, 15066597, 15132390, 15198183, 15263976, 15329769, 15395562, 15461355, 15527148, 15592941, 15658734, 15724527, 15790320, 15856113, 15921906, 15987699, 16053492, 16119285, 16185078, 16250871, 16316664, 16382457, 16448250, 16514043, 16579836, 16645629, 16711422, 16448250] ("256 gray scale") u32[] [16448250, 16711422, 16645629, 16579836, 16514043, 16448250, 16382457, 16316664, 16250871, 16185078, 16119285, 16053492, 15987699, 15921906, 15856113, 15790320, 15724527, 15658734, 15592941, 15527148, 15461355, 15395562, 15329769, 15263976, 15198183, 15132390, 15066597, 15000804, 14935011, 14869218, 14803425, 14737632, 14671839, 14606046, 14540253, 14474460, 14408667, 14342874, 14277081, 14211288, 14145495, 14079702, 14013909, 13948116, 13882323, 13816530, 13750737, 13684944, 13619151, 13553358, 13487565, 13421772, 13355979, 13290186, 13224393, 13158600, 13092807, 13027014, 12961221, 12895428, 12829635, 12763842, 12698049, 12632256, 12566463, 12500670, 12434877, 12369084, 12303291, 12237498, 12171705, 12105912, 12040119, 11974326, 11908533, 11842740, 11776947, 11711154, 11645361, 11579568, 11513775, 11447982, 11382189, 11316396, 11250603, 11184810, 11119017, 11053224, 10987431, 10921638, 10855845, 10790052, 10724259, 10658466, 10592673, 10526880, 10461087, 10395294, 10329501, 10263708, 10197915, 10132122, 10066329, 10000536, 9934743, 9868950, 9803157, 9737364, 9671571, 9605778, 9539985, 9474192, 9408399, 9342606, 9276813, 9211020, 9145227, 9079434, 9013641, 8947848, 8882055, 8816262, 8750469, 8684676, 8618883, 8553090, 8487297, 8421504, 8355711, 8289918, 8224125, 8158332, 8092539, 8026746, 7960953, 7895160, 7829367, 7763574, 7697781, 7631988, 7566195, 7500402, 7434609, 7368816, 7303023, 7237230, 7171437, 7105644, 7039851, 6974058, 6908265, 6842472, 6776679, 6710886, 6645093, 6579300, 6513507, 6447714, 6381921, 6316128, 6250335, 6184542, 6118749, 6052956, 5987163, 5921370, 5855577, 5789784, 5723991, 5658198, 5592405, 5526612, 5460819, 5395026, 5329233, 5263440, 5197647, 5131854, 5066061, 5000268, 4934475, 4868682, 4802889, 4737096, 4671303, 4605510, 4539717, 4473924, 4408131, 4342338, 4276545, 4210752, 4144959, 4079166, 4013373, 3947580, 3881787, 3815994, 3750201, 3684408, 3618615, 3552822, 3487029, 3421236, 3355443, 3289650, 3223857, 3158064, 3092271, 3026478, 2960685, 2894892, 2829099, 2763306, 2697513, 2631720, 2565927, 2500134, 2434341, 2368548, 2302755, 2236962, 2171169, 2105376, 2039583, 1973790, 1907997, 1842204, 1776411, 1710618, 1644825, 1579032, 1513239, 1447446, 1381653, 1315860, 1250067, 1184274, 1118481, 1052688, 986895, 921102, 855309, 789516, 723723, 657930, 592137, 526344, 460551, 394758, 328965, 263172, 197379, 131586, 65793, 16777222] ("256 gray scale inverse")] -> _
        frame False {
        }
        frame True {
        }
      }
      n76 = To Unsigned Word Integer(number=w160) -> (unsigned 16bit integer=w48:u16)
      n77 = local read "Det A I/O"() -> (w121:tag)
      n78 = Build Array(w115, w114) -> (w113:tag[])
      n79 = In Range and Coerce(upper limit=w48, x=w48, lower limit=u16 1) -> (coerced(x)=w47:u16)  [unwired: 1 out]
      n80 = Unbundle By Name("FIB Para") -> ("Z-step (nm)"=→"Z-step (nm)":dbl)  [unwired: 2 out]
      n81 = local read "Inverse B"() -> (w176:bool)
      n82 = call <vilib>:"DAQmx Flatten Channel String.vi"("names in"=w113) -> ("names out"=w116:string, "error out"=w54:errorcluster)  [unwired: 1 in, 12 out]
      n83 = local write "Decimating factor"(w47) -> ()
      n84 = call-poly <vilib>:"DAQmx Create Virtual Channel.vi"("physical channels"=w116, "error in"=w54) -> ("task out"=w125:refnum<k21>, "error out"=w120:errorcluster)  [unwired: 7 in, 5 out]
      n85 = call-poly <vilib>:"DAQmx Create Virtual Channel.vi"("physical channels"=w121) -> ("task out"=w122:refnum<k21>, "error out"=w117:errorcluster)  [unwired: 8 in, 5 out]
      n86 = case shown="False" w176 {
        tunnel: [u32[] [16777222, 65793, 131586, 197379, 263172, 328965, 394758, 460551, 526344, 592137, 657930, 723723, 789516, 855309, 921102, 986895, 1052688, 1118481, 1184274, 1250067, 1315860, 1381653, 1447446, 1513239, 1579032, 1644825, 1710618, 1776411, 1842204, 1907997, 1973790, 2039583, 2105376, 2171169, 2236962, 2302755, 2368548, 2434341, 2500134, 2565927, 2631720, 2697513, 2763306, 2829099, 2894892, 2960685, 3026478, 3092271, 3158064, 3223857, 3289650, 3355443, 3421236, 3487029, 3552822, 3618615, 3684408, 3750201, 3815994, 3881787, 3947580, 4013373, 4079166, 4144959, 4210752, 4276545, 4342338, 4408131, 4473924, 4539717, 4605510, 4671303, 4737096, 4802889, 4868682, 4934475, 5000268, 5066061, 5131854, 5197647, 5263440, 5329233, 5395026, 5460819, 5526612, 5592405, 5658198, 5723991, 5789784, 5855577, 5921370, 5987163, 6052956, 6118749, 6184542, 6250335, 6316128, 6381921, 6447714, 6513507, 6579300, 6645093, 6710886, 6776679, 6842472, 6908265, 6974058, 7039851, 7105644, 7171437, 7237230, 7303023, 7368816, 7434609, 7500402, 7566195, 7631988, 7697781, 7763574, 7829367, 7895160, 7960953, 8026746, 8092539, 8158332, 8224125, 8289918, 8355711, 8421504, 8487297, 8553090, 8618883, 8684676, 8750469, 8816262, 8882055, 8947848, 9013641, 9079434, 9145227, 9211020, 9276813, 9342606, 9408399, 9474192, 9539985, 9605778, 9671571, 9737364, 9803157, 9868950, 9934743, 10000536, 10066329, 10132122, 10197915, 10263708, 10329501, 10395294, 10461087, 10526880, 10592673, 10658466, 10724259, 10790052, 10855845, 10921638, 10987431, 11053224, 11119017, 11184810, 11250603, 11316396, 11382189, 11447982, 11513775, 11579568, 11645361, 11711154, 11776947, 11842740, 11908533, 11974326, 12040119, 12105912, 12171705, 12237498, 12303291, 12369084, 12434877, 12500670, 12566463, 12632256, 12698049, 12763842, 12829635, 12895428, 12961221, 13027014, 13092807, 13158600, 13224393, 13290186, 13355979, 13421772, 13487565, 13553358, 13619151, 13684944, 13750737, 13816530, 13882323, 13948116, 14013909, 14079702, 14145495, 14211288, 14277081, 14342874, 14408667, 14474460, 14540253, 14606046, 14671839, 14737632, 14803425, 14869218, 14935011, 15000804, 15066597, 15132390, 15198183, 15263976, 15329769, 15395562, 15461355, 15527148, 15592941, 15658734, 15724527, 15790320, 15856113, 15921906, 15987699, 16053492, 16119285, 16185078, 16250871, 16316664, 16382457, 16448250, 16514043, 16579836, 16645629, 16711422, 16448250] ("256 gray scale") u32[] [16448250, 16711422, 16645629, 16579836, 16514043, 16448250, 16382457, 16316664, 16250871, 16185078, 16119285, 16053492, 15987699, 15921906, 15856113, 15790320, 15724527, 15658734, 15592941, 15527148, 15461355, 15395562, 15329769, 15263976, 15198183, 15132390, 15066597, 15000804, 14935011, 14869218, 14803425, 14737632, 14671839, 14606046, 14540253, 14474460, 14408667, 14342874, 14277081, 14211288, 14145495, 14079702, 14013909, 13948116, 13882323, 13816530, 13750737, 13684944, 13619151, 13553358, 13487565, 13421772, 13355979, 13290186, 13224393, 13158600, 13092807, 13027014, 12961221, 12895428, 12829635, 12763842, 12698049, 12632256, 12566463, 12500670, 12434877, 12369084, 12303291, 12237498, 12171705, 12105912, 12040119, 11974326, 11908533, 11842740, 11776947, 11711154, 11645361, 11579568, 11513775, 11447982, 11382189, 11316396, 11250603, 11184810, 11119017, 11053224, 10987431, 10921638, 10855845, 10790052, 10724259, 10658466, 10592673, 10526880, 10461087, 10395294, 10329501, 10263708, 10197915, 10132122, 10066329, 10000536, 9934743, 9868950, 9803157, 9737364, 9671571, 9605778, 9539985, 9474192, 9408399, 9342606, 9276813, 9211020, 9145227, 9079434, 9013641, 8947848, 8882055, 8816262, 8750469, 8684676, 8618883, 8553090, 8487297, 8421504, 8355711, 8289918, 8224125, 8158332, 8092539, 8026746, 7960953, 7895160, 7829367, 7763574, 7697781, 7631988, 7566195, 7500402, 7434609, 7368816, 7303023, 7237230, 7171437, 7105644, 7039851, 6974058, 6908265, 6842472, 6776679, 6710886, 6645093, 6579300, 6513507, 6447714, 6381921, 6316128, 6250335, 6184542, 6118749, 6052956, 5987163, 5921370, 5855577, 5789784, 5723991, 5658198, 5592405, 5526612, 5460819, 5395026, 5329233, 5263440, 5197647, 5131854, 5066061, 5000268, 4934475, 4868682, 4802889, 4737096, 4671303, 4605510, 4539717, 4473924, 4408131, 4342338, 4276545, 4210752, 4144959, 4079166, 4013373, 3947580, 3881787, 3815994, 3750201, 3684408, 3618615, 3552822, 3487029, 3421236, 3355443, 3289650, 3223857, 3158064, 3092271, 3026478, 2960685, 2894892, 2829099, 2763306, 2697513, 2631720, 2565927, 2500134, 2434341, 2368548, 2302755, 2236962, 2171169, 2105376, 2039583, 1973790, 1907997, 1842204, 1776411, 1710618, 1644825, 1579032, 1513239, 1447446, 1381653, 1315860, 1250067, 1184274, 1118481, 1052688, 986895, 921102, 855309, 789516, 723723, 657930, 592137, 526344, 460551, 394758, 328965, 263172, 197379, 131586, 65793, 16777222] ("256 gray scale inverse")] -> _
        frame False {
        }
        frame True {
        }
      }
      n87 = property class="DAQmx Timing"(reference=w125, error in=w120) -> (reference out=w124:refnum<k21>, error out=w119:errorcluster, "SampClk.MaxRate"=w110:dbl)
      n88 = property class="DAQmx Timing"(reference=w122, error in=w117) -> (reference out=w123:refnum<k21>, error out=w118:errorcluster, "SampClk.MaxRate"=w111:dbl)
      n89 = local read "Inverse C"() -> (w177:bool)
      n90 = case shown="False" w177 {
        tunnel: [u32[] [16777222, 65793, 131586, 197379, 263172, 328965, 394758, 460551, 526344, 592137, 657930, 723723, 789516, 855309, 921102, 986895, 1052688, 1118481, 1184274, 1250067, 1315860, 1381653, 1447446, 1513239, 1579032, 1644825, 1710618, 1776411, 1842204, 1907997, 1973790, 2039583, 2105376, 2171169, 2236962, 2302755, 2368548, 2434341, 2500134, 2565927, 2631720, 2697513, 2763306, 2829099, 2894892, 2960685, 3026478, 3092271, 3158064, 3223857, 3289650, 3355443, 3421236, 3487029, 3552822, 3618615, 3684408, 3750201, 3815994, 3881787, 3947580, 4013373, 4079166, 4144959, 4210752, 4276545, 4342338, 4408131, 4473924, 4539717, 4605510, 4671303, 4737096, 4802889, 4868682, 4934475, 5000268, 5066061, 5131854, 5197647, 5263440, 5329233, 5395026, 5460819, 5526612, 5592405, 5658198, 5723991, 5789784, 5855577, 5921370, 5987163, 6052956, 6118749, 6184542, 6250335, 6316128, 6381921, 6447714, 6513507, 6579300, 6645093, 6710886, 6776679, 6842472, 6908265, 6974058, 7039851, 7105644, 7171437, 7237230, 7303023, 7368816, 7434609, 7500402, 7566195, 7631988, 7697781, 7763574, 7829367, 7895160, 7960953, 8026746, 8092539, 8158332, 8224125, 8289918, 8355711, 8421504, 8487297, 8553090, 8618883, 8684676, 8750469, 8816262, 8882055, 8947848, 9013641, 9079434, 9145227, 9211020, 9276813, 9342606, 9408399, 9474192, 9539985, 9605778, 9671571, 9737364, 9803157, 9868950, 9934743, 10000536, 10066329, 10132122, 10197915, 10263708, 10329501, 10395294, 10461087, 10526880, 10592673, 10658466, 10724259, 10790052, 10855845, 10921638, 10987431, 11053224, 11119017, 11184810, 11250603, 11316396, 11382189, 11447982, 11513775, 11579568, 11645361, 11711154, 11776947, 11842740, 11908533, 11974326, 12040119, 12105912, 12171705, 12237498, 12303291, 12369084, 12434877, 12500670, 12566463, 12632256, 12698049, 12763842, 12829635, 12895428, 12961221, 13027014, 13092807, 13158600, 13224393, 13290186, 13355979, 13421772, 13487565, 13553358, 13619151, 13684944, 13750737, 13816530, 13882323, 13948116, 14013909, 14079702, 14145495, 14211288, 14277081, 14342874, 14408667, 14474460, 14540253, 14606046, 14671839, 14737632, 14803425, 14869218, 14935011, 15000804, 15066597, 15132390, 15198183, 15263976, 15329769, 15395562, 15461355, 15527148, 15592941, 15658734, 15724527, 15790320, 15856113, 15921906, 15987699, 16053492, 16119285, 16185078, 16250871, 16316664, 16382457, 16448250, 16514043, 16579836, 16645629, 16711422, 16448250] ("256 gray scale") u32[] [16448250, 16711422, 16645629, 16579836, 16514043, 16448250, 16382457, 16316664, 16250871, 16185078, 16119285, 16053492, 15987699, 15921906, 15856113, 15790320, 15724527, 15658734, 15592941, 15527148, 15461355, 15395562, 15329769, 15263976, 15198183, 15132390, 15066597, 15000804, 14935011, 14869218, 14803425, 14737632, 14671839, 14606046, 14540253, 14474460, 14408667, 14342874, 14277081, 14211288, 14145495, 14079702, 14013909, 13948116, 13882323, 13816530, 13750737, 13684944, 13619151, 13553358, 13487565, 13421772, 13355979, 13290186, 13224393, 13158600, 13092807, 13027014, 12961221, 12895428, 12829635, 12763842, 12698049, 12632256, 12566463, 12500670, 12434877, 12369084, 12303291, 12237498, 12171705, 12105912, 12040119, 11974326, 11908533, 11842740, 11776947, 11711154, 11645361, 11579568, 11513775, 11447982, 11382189, 11316396, 11250603, 11184810, 11119017, 11053224, 10987431, 10921638, 10855845, 10790052, 10724259, 10658466, 10592673, 10526880, 10461087, 10395294, 10329501, 10263708, 10197915, 10132122, 10066329, 10000536, 9934743, 9868950, 9803157, 9737364, 9671571, 9605778, 9539985, 9474192, 9408399, 9342606, 9276813, 9211020, 9145227, 9079434, 9013641, 8947848, 8882055, 8816262, 8750469, 8684676, 8618883, 8553090, 8487297, 8421504, 8355711, 8289918, 8224125, 8158332, 8092539, 8026746, 7960953, 7895160, 7829367, 7763574, 7697781, 7631988, 7566195, 7500402, 7434609, 7368816, 7303023, 7237230, 7171437, 7105644, 7039851, 6974058, 6908265, 6842472, 6776679, 6710886, 6645093, 6579300, 6513507, 6447714, 6381921, 6316128, 6250335, 6184542, 6118749, 6052956, 5987163, 5921370, 5855577, 5789784, 5723991, 5658198, 5592405, 5526612, 5460819, 5395026, 5329233, 5263440, 5197647, 5131854, 5066061, 5000268, 4934475, 4868682, 4802889, 4737096, 4671303, 4605510, 4539717, 4473924, 4408131, 4342338, 4276545, 4210752, 4144959, 4079166, 4013373, 3947580, 3881787, 3815994, 3750201, 3684408, 3618615, 3552822, 3487029, 3421236, 3355443, 3289650, 3223857, 3158064, 3092271, 3026478, 2960685, 2894892, 2829099, 2763306, 2697513, 2631720, 2565927, 2500134, 2434341, 2368548, 2302755, 2236962, 2171169, 2105376, 2039583, 1973790, 1907997, 1842204, 1776411, 1710618, 1644825, 1579032, 1513239, 1447446, 1381653, 1315860, 1250067, 1184274, 1118481, 1052688, 986895, 921102, 855309, 789516, 723723, 657930, 592137, 526344, 460551, 394758, 328965, 263172, 197379, 131586, 65793, 16777222] ("256 gray scale inverse")] -> _
        frame False {
        }
        frame True {
        }
      }
      n91 = local write "AO SampClk.MaxRate"(w110) -> ()
      n92 = local write "AI SampClk.MaxRate"(w111) -> ()
      n93 = call <vilib>:"DAQmx Clear Task.vi"("task in"=w124, "error in"=w119) -> ()  [unwired: 14 out]
      n94 = call <vilib>:"DAQmx Clear Task.vi"("task in"=w123, "error in"=w118) -> ()  [unwired: 14 out]
      n95 = local read "Inverse D"() -> (w178:bool)
      n96 = case shown="False" w178 {
        tunnel: [u32[] [16777222, 65793, 131586, 197379, 263172, 328965, 394758, 460551, 526344, 592137, 657930, 723723, 789516, 855309, 921102, 986895, 1052688, 1118481, 1184274, 1250067, 1315860, 1381653, 1447446, 1513239, 1579032, 1644825, 1710618, 1776411, 1842204, 1907997, 1973790, 2039583, 2105376, 2171169, 2236962, 2302755, 2368548, 2434341, 2500134, 2565927, 2631720, 2697513, 2763306, 2829099, 2894892, 2960685, 3026478, 3092271, 3158064, 3223857, 3289650, 3355443, 3421236, 3487029, 3552822, 3618615, 3684408, 3750201, 3815994, 3881787, 3947580, 4013373, 4079166, 4144959, 4210752, 4276545, 4342338, 4408131, 4473924, 4539717, 4605510, 4671303, 4737096, 4802889, 4868682, 4934475, 5000268, 5066061, 5131854, 5197647, 5263440, 5329233, 5395026, 5460819, 5526612, 5592405, 5658198, 5723991, 5789784, 5855577, 5921370, 5987163, 6052956, 6118749, 6184542, 6250335, 6316128, 6381921, 6447714, 6513507, 6579300, 6645093, 6710886, 6776679, 6842472, 6908265, 6974058, 7039851, 7105644, 7171437, 7237230, 7303023, 7368816, 7434609, 7500402, 7566195, 7631988, 7697781, 7763574, 7829367, 7895160, 7960953, 8026746, 8092539, 8158332, 8224125, 8289918, 8355711, 8421504, 8487297, 8553090, 8618883, 8684676, 8750469, 8816262, 8882055, 8947848, 9013641, 9079434, 9145227, 9211020, 9276813, 9342606, 9408399, 9474192, 9539985, 9605778, 9671571, 9737364, 9803157, 9868950, 9934743, 10000536, 10066329, 10132122, 10197915, 10263708, 10329501, 10395294, 10461087, 10526880, 10592673, 10658466, 10724259, 10790052, 10855845, 10921638, 10987431, 11053224, 11119017, 11184810, 11250603, 11316396, 11382189, 11447982, 11513775, 11579568, 11645361, 11711154, 11776947, 11842740, 11908533, 11974326, 12040119, 12105912, 12171705, 12237498, 12303291, 12369084, 12434877, 12500670, 12566463, 12632256, 12698049, 12763842, 12829635, 12895428, 12961221, 13027014, 13092807, 13158600, 13224393, 13290186, 13355979, 13421772, 13487565, 13553358, 13619151, 13684944, 13750737, 13816530, 13882323, 13948116, 14013909, 14079702, 14145495, 14211288, 14277081, 14342874, 14408667, 14474460, 14540253, 14606046, 14671839, 14737632, 14803425, 14869218, 14935011, 15000804, 15066597, 15132390, 15198183, 15263976, 15329769, 15395562, 15461355, 15527148, 15592941, 15658734, 15724527, 15790320, 15856113, 15921906, 15987699, 16053492, 16119285, 16185078, 16250871, 16316664, 16382457, 16448250, 16514043, 16579836, 16645629, 16711422, 16448250] ("256 gray scale") u32[] [16448250, 16711422, 16645629, 16579836, 16514043, 16448250, 16382457, 16316664, 16250871, 16185078, 16119285, 16053492, 15987699, 15921906, 15856113, 15790320, 15724527, 15658734, 15592941, 15527148, 15461355, 15395562, 15329769, 15263976, 15198183, 15132390, 15066597, 15000804, 14935011, 14869218, 14803425, 14737632, 14671839, 14606046, 14540253, 14474460, 14408667, 14342874, 14277081, 14211288, 14145495, 14079702, 14013909, 13948116, 13882323, 13816530, 13750737, 13684944, 13619151, 13553358, 13487565, 13421772, 13355979, 13290186, 13224393, 13158600, 13092807, 13027014, 12961221, 12895428, 12829635, 12763842, 12698049, 12632256, 12566463, 12500670, 12434877, 12369084, 12303291, 12237498, 12171705, 12105912, 12040119, 11974326, 11908533, 11842740, 11776947, 11711154, 11645361, 11579568, 11513775, 11447982, 11382189, 11316396, 11250603, 11184810, 11119017, 11053224, 10987431, 10921638, 10855845, 10790052, 10724259, 10658466, 10592673, 10526880, 10461087, 10395294, 10329501, 10263708, 10197915, 10132122, 10066329, 10000536, 9934743, 9868950, 9803157, 9737364, 9671571, 9605778, 9539985, 9474192, 9408399, 9342606, 9276813, 9211020, 9145227, 9079434, 9013641, 8947848, 8882055, 8816262, 8750469, 8684676, 8618883, 8553090, 8487297, 8421504, 8355711, 8289918, 8224125, 8158332, 8092539, 8026746, 7960953, 7895160, 7829367, 7763574, 7697781, 7631988, 7566195, 7500402, 7434609, 7368816, 7303023, 7237230, 7171437, 7105644, 7039851, 6974058, 6908265, 6842472, 6776679, 6710886, 6645093, 6579300, 6513507, 6447714, 6381921, 6316128, 6250335, 6184542, 6118749, 6052956, 5987163, 5921370, 5855577, 5789784, 5723991, 5658198, 5592405, 5526612, 5460819, 5395026, 5329233, 5263440, 5197647, 5131854, 5066061, 5000268, 4934475, 4868682, 4802889, 4737096, 4671303, 4605510, 4539717, 4473924, 4408131, 4342338, 4276545, 4210752, 4144959, 4079166, 4013373, 3947580, 3881787, 3815994, 3750201, 3684408, 3618615, 3552822, 3487029, 3421236, 3355443, 3289650, 3223857, 3158064, 3092271, 3026478, 2960685, 2894892, 2829099, 2763306, 2697513, 2631720, 2565927, 2500134, 2434341, 2368548, 2302755, 2236962, 2171169, 2105376, 2039583, 1973790, 1907997, 1842204, 1776411, 1710618, 1644825, 1579032, 1513239, 1447446, 1381653, 1315860, 1250067, 1184274, 1118481, 1052688, 986895, 921102, 855309, 789516, 723723, 657930, 592137, 526344, 460551, 394758, 328965, 263172, 197379, 131586, 65793, 16777222] ("256 gray scale inverse")] -> _
        frame False {
        }
        frame True {
        }
      }
      n97 = local read "AO SampClk.MaxRate"() -> (w128:dbl)
      n98 = local read "Oversampling"() -> (w132:u16)
      n99 = local read "AI SampClk.MaxRate"() -> (w126:dbl)
      n100 = local read "Scan rate (Hz)"() -> (w135:u32)
      n101 = local read "Detector A"() -> (w139:bool)
      n102 = local read "Detector B"() -> (w138:bool)
      n103 = local read "Detector C"() -> (w140:bool)
      n104 = local read "Detector D"() -> (w141:bool)
      n105 = Boolean To (0,1)(Boolean=w139) -> (0, 1=w136:i16)
      n106 = Boolean To (0,1)(Boolean=w138) -> (0, 1=w137:i16)
      n107 = Boolean To (0,1)(Boolean=w140) -> (0, 1=w142:i16)
      n108 = Boolean To (0,1)(Boolean=w141) -> (0, 1=w143:i16)
      n109 = Divide(x=w126, y=w135) -> (x/y=w130:dbl)
      n110 = Compound Arithmetic op=ADD(w136, w137, w142, w143) -> (w144:i16)
      n111 = In Range and Coerce(upper limit=w128, x=w135, lower limit=u32 100) -> (coerced(x)=w127:dbl)  [unwired: 1 out]
      n112 = In Range and Coerce(upper limit=w130, x=w132, lower limit=u8 1) -> (coerced(x)=w131:dbl)  [unwired: 1 out]
      n113 = local write "Detector number"(w144) -> ()
      n114 = Round Toward -Infinity(1:w131) -> (0:w134:dbl)
      n115 = local write "Scan rate (Hz)"(w127) -> ()
      n116 = local write "Oversampling"(w134) -> ()
    }
    frame #1 {
      w231 = T12 3 items=["no dialog", "OK message", "continue or stop message", "OK message + warnings", "continue/stop + warnings"] ("type of dialog (OK msg:1)")
      w235 = 0 items=["one channel for each line", "one channel for all lines"] ("line grouping")
      n117 = local read "COM port"() -> (w224:refnum<visa-resource-name>)
      n118 = local read "X center"() -> (w238:dbl)
      n119 = local read "X size (V)"() -> (w239:dbl)
      n120 = local read "Y center"() -> (w241:dbl)
      n121 = local read "Y size (V)"() -> (w242:dbl)
      n122 = expression code="x/2"(w239) -> (w240:dbl)
      n123 = expression code="x/2"(w242) -> (w243:dbl)
      n124 = call "Remcon32 command.vi"("Initialization"=TRUE, "SEM command"="frez" ("write buffer"), "COM port in"=w224) -> ("error out"=w188:errorcluster, "COM port out"=w190:refnum<visa-resource-name>)  [unwired: 2 in, 5 out]
      n125 = Subtract(x=w238, y=w240) -> (x-y=→"X min set":dbl)
      n126 = Add(x=w238, y=w240) -> (x+y=→"X max set":dbl)
      n127 = Subtract(x=w241, y=w243) -> (x-y=→"Y min set":dbl)
      n128 = Add(x=w241, y=w243) -> (x+y=→"Y max set":dbl)
      n129 = local read "Set WD"() -> (w209:bool)
      n130 = call "Remcon32 command.vi"("error in"=w188, "SEM command"="edx 1" ("write buffer"), "COM port in"=w190) -> ("error out"=w187:errorcluster, "COM port out"=w189:refnum<visa-resource-name>)  [unwired: 2 in, 5 out]
      n131 = stacked-sequence {
        tunnel: w189 -> [w334]
        tunnel: w187 -> [w333]
        tunnel: [w334] -> w221
        tunnel: [w333] -> w220
        frame #0 {
        }
      }
      n132 = local read "Detector FIB-NI auto switch"() -> (w227:tag)
      n133 = local write "Total lines scanned"(0 ("Read line")) -> ()
      n134 = local read "Set Mag"() -> (w208:bool)
      n135 = local read "Set Det A para"() -> (w210:bool)
      n136 = call "FIB mode.vi"("error in"=w220, "Iterations"=u32 1, "FIB mode"=T10."SEM", "COM port in"=w221) -> ("error out"=w211:errorcluster, "COM port out"=w212:refnum<visa-resource-name>)  [unwired: 2 in, 4 out]
      n137 = call-poly <vilib>:"DAQmx Create Virtual Channel.vi"("lines"=w227, "line grouping"=w235) -> ("task out"=w237:refnum<k21>, "error out"=w236:errorcluster)  [unwired: 3 in, 9 out]
      n138 = call <vilib>:"DAQmx Start Task.vi"("task/channels in"=w237, "error in"=w236) -> ("task out"=w234:refnum<k21>, "error out"=w233:errorcluster)  [unwired: 12 out]
      n139 = case shown="True" w210 {
        tunnel: w212 -> [w286 w290]
        tunnel: w211 -> [w285 w289]
        tunnel: [w286 w298] -> w205
        tunnel: [w285 w297] -> w203
        frame False {
        }
        frame True {
          n140 = local read "Brightness A"() -> (w287:dbl)
          n141 = Format Into String(format string="brgt %g", w287) -> (resulting string=w293:string)  [unwired: 2 in, 1 out]
          n142 = call "Remcon32 command.vi"("error in"=w289, "SEM command"=w293, "COM port in"=w290) -> ("error out"=w291:errorcluster, "COM port out"=w292:refnum<visa-resource-name>)  [unwired: 2 in, 5 out]
          n143 = local read "Contrast A"() -> (w288:dbl)
          n144 = Format Into String(format string="crst %g", w288) -> (resulting string=w295:string)  [unwired: 2 in, 1 out]
          n145 = call "Remcon32 command.vi"("error in"=w291, "SEM command"=w295, "COM port in"=w292) -> ("error out"=w297:errorcluster, "COM port out"=w298:refnum<visa-resource-name>)  [unwired: 2 in, 5 out]
        }
      }
      n146 = local read "X size (V)"() -> (w215:dbl)
      n147 = local read "X resolution"() -> (w207:u32)
      n148 = call-poly <vilib>:"DAQmx Write.vi"("task/channels in"=w234, "data"=TRUE, "error in"=w233) -> ("task out"=w229:refnum<k21>, "error out"=w228:errorcluster)  [unwired: 1 in, 10 out]
      n149 = To Double Precision Float(number=w207) -> (double precision float=w213:dbl)
      n150 = expression code="x/20*1024"(w215) -> (w214:dbl)
      n151 = call <vilib>:"DAQmx Clear Task.vi"("task in"=w229, "error in"=w228) -> ("error out"=w230:errorcluster)  [unwired: 13 out]
      n152 = call <vilib>:"Simple Error Handler.vi"("type of dialog (OK msg:1)"=w231, "error in (no error)"=w230) -> ()  [unwired: 8 out]
      n153 = local read "HW Config"() -> (w200:T9)
      n154 = Unbundle By Name(w200) -> ("Machine Type"=w199:u8)
      n155 = local read "Set X stig"() -> (w206:bool)
      n156 = local read "GetInfo"() -> (w201:bool)
      n157 = case shown="0, Default" w199 {
        tunnel: [FALSE ("Initialization") TRUE ("Initialization")] -> w198
        frame 0, Default {
        }
        frame 1 {
        }
      }
      n158 = case shown="True" w206 {
        tunnel: [w276 w284] -> w204
        tunnel: [w275 w283] -> w202
        tunnel: w205 -> [w276 w282]
        tunnel: w203 -> [w275 w281]
        frame False {
        }
        frame True {
          n159 = local read "X stig"() -> (w278:dbl)
          n160 = local read "Y stig"() -> (w280:dbl)
          n161 = Format Into String(format string="stim %g %g", w278, w280) -> (resulting string=w277:string)  [unwired: 2 in, 1 out]
          n162 = call "Remcon32 command.vi"("error in"=w281, "SEM command"=w277, "COM port in"=w282) -> ("error out"=w283:errorcluster, "COM port out"=w284:refnum<visa-resource-name>)  [unwired: 2 in, 5 out]
        }
      }
      n163 = case shown="True" w209 {
        tunnel: w204 -> [w322 w332]
        tunnel: w202 -> [w321 w331]
        tunnel: [w322 w329] -> w219
        tunnel: [w321 w327] -> w217
        frame False {
        }
        frame True {
          n164 = local read "WD"() -> (w325:dbl)
          n165 = call "Remcon32 command.vi"("error in"=w331, "SEM command"="fblk 1", "COM port in"=w332) -> ("error out"=w328:errorcluster, "COM port out"=w330:refnum<visa-resource-name>)  [unwired: 2 in, 5 out]
          n166 = Format Into String(format string="focs %g", w325) -> (resulting string=w323:string)  [unwired: 2 in, 1 out]
          n167 = call "Remcon32 command.vi"("error in"=w328, "SEM command"=w323, "COM port in"=w330) -> ("error out"=w327:errorcluster, "COM port out"=w329:refnum<visa-resource-name>)  [unwired: 2 in, 5 out]
        }
      }
      n168 = case shown="True" w208 {
        tunnel: w219 -> [w307 w311]
        tunnel: [w307 w317] -> w218
        tunnel: w217 -> [w306 w310]
        tunnel: [w306 w316] -> w216
        tunnel: w213 -> [w302 w314]
        tunnel: w214 -> [w301 w313]
        tunnel: [w300 w309] -> w197
        tunnel: [w299 w308] -> w196
        frame False {
          n169 = local read "Pixel size (nm)"() -> (w299:dbl)
          n170 = Divide(x=111652.0, y=w299) -> (x/y=w304:dbl)
          n171 = Multiply(x=w301, y=w304) -> (x*y=w305:dbl)
          n172 = Divide(x=w305, y=w302) -> (x/y=w300:dbl)
        }
        frame True {
          n173 = local read "Pixel size (nm)"() -> (w308:dbl)
          n174 = Divide(x=111652.0, y=w308) -> (x/y=w315:dbl)
          n175 = Multiply(x=w313, y=w315) -> (x*y=w320:dbl)
          n176 = Divide(x=w320, y=w314) -> (x/y=w309:dbl)
          n177 = Format Into String(format string="mag %g", w309) -> (resulting string=w318:string)  [unwired: 2 in, 1 out]
          n178 = call "Remcon32 command.vi"("error in"=w310, "SEM command"=w318, "COM port in"=w311) -> ("error out"=w316:errorcluster, "COM port out"=w317:refnum<visa-resource-name>)  [unwired: 2 in, 5 out]
        }
      }
      n179 = case shown="True" w201 {
        tunnel: [w257 w274] -> w193
        tunnel: [w256 w273] -> w192
        tunnel: w218 -> [w257 w270]
        tunnel: w216 -> [w256 w269]
        tunnel: w214 -> [_ w268]
        tunnel: w213 -> [_ w267]
        tunnel: w198 -> [_ w258]
        tunnel: w197 -> [w253 _]
        tunnel: w196 -> [w252 _]
        frame False {
          n180 = local read "SEM parameters"() -> (w255:T2)
          n181 = Bundle By Name(cluster=w255, "Magnification"=w253, "Pixel size"=w252) -> (w254:T2)
          n182 = local write "SEM parameters"(w254) -> ()
          n183 = Wait (ms)(milliseconds to wait=u32 100) -> ()  [unwired: 1 out]
        }
        frame True {
          w259 = FALSE ("Initialization")
          n184 = call "Read Zeiss Parameters.vi"("Close session"=w259, "Initialization"=w259, "error in (no error)"=w269, "FIB"=w258, "COM port in"=w270) -> ("error out"=w273:errorcluster, "FIB parameters"=→"FIB parameters":T3, "SEM parameters"=w261:T2, "COM port out"=w274:refnum<visa-resource-name>)  [unwired: 3 out]
          n185 = local read "Detector B name"() -> (w264:string)
          n186 = local read "Brightness B"() -> (w265:dbl)
          n187 = local read "Contrast B"() -> (w266:dbl)
          n188 = Unbundle By Name(w261) -> ("Pixel size"=w260:sgl)
          n189 = Multiply(x=w268, y=w260) -> (x*y=w272:dbl)
          n190 = Divide(x=w272, y=w267) -> (x/y=w271:dbl)
          n191 = Bundle By Name(cluster=w261, "Detector B"=w264, "Brightness B"=w265, "Contrast B"=w266, "Pixel size"=w271) -> (→"SEM parameters":T2)
        }
      }
      n192 = call "Remcon32 command.vi"("Close session"=TRUE, "error in"=w192, "SEM command"="edx 1" ("write buffer"), "COM port in"=w193) -> ()  [unwired: 1 in, 7 out]
    }
    frame #2 {
      w375 = 1 ("dimension size")
      w491 = T12 3 items=["no dialog", "OK message", "continue or stop message", "OK message + warnings", "continue/stop + warnings"] ("type of dialog (OK msg:1)")
      w489 = 10280 items=["Rising"=10280, "Falling"=10171] ("edge")
      w487 = 10123 items=["Finite Samples"=10178, "Continuous Samples"=10123, "Hardware Timed Single Point"=12522] ("sample mode")
      w499 = 10158 items=["Allow Regeneration"=10097, "Do Not Allow Regeneration"=10158] ("RegenMode")
      w500 = 10178 items=["Finite Samples"=10178, "Continuous Samples"=10123, "Hardware Timed Single Point"=12522] ("sample mode")
      n193 = local read "Det min (V)"() -> (w382:dbl)
      n194 = local read "Det max (V)"() -> (w383:dbl)
      n195 = local read "Decimating factor"() -> (w429:u16)
      n196 = local read "Y resolution"() -> (w430:u32)
      n197 = local read "X resolution"() -> (w431:u32)
      n198 = local read "Save"() -> (w390:bool)
      n199 = local read "SEM X coil"() -> (w399:tag)
      n200 = local read "Oversampling"() -> (w393:u16)
      n201 = local read "Detector A"() -> (w397:bool)
      n202 = local read "Detector C"() -> (w395:bool)
      n203 = local read "Detector C"() -> (w360:bool)
      n204 = local read "Detector A"() -> (w377:bool)
      n205 = local read "Display"() -> (w378:bool)
      n206 = local read "Detector B"() -> (w367:bool)
      n207 = local read "Display"() -> (w366:bool)
      n208 = local read "Display"() -> (w361:bool)
      n209 = local read "Detector D"() -> (w358:bool)
      n210 = local read "Display"() -> (w357:bool)
      n211 = case shown="True" w397 {
        tunnel: [_ w1592] -> w452
        tunnel: [_ w1591] -> w451
        tunnel: w382 -> [w1587 w1589]
        tunnel: w383 -> [w1586 w1588]
        tunnel: [w1587 w1589] -> w385
        tunnel: [w1586 w1588] -> w384
        frame False {
        }
        frame True {
          n212 = local read "Det A I/O"() -> (w1590:tag)
          n213 = call-poly <vilib>:"DAQmx Create Virtual Channel.vi"("maximum value"=w1588, "minimum value"=w1589, "physical channels"=w1590) -> ("task out"=w1592:refnum<k21>, "error out"=w1591:errorcluster)  [unwired: 6 in, 5 out]
        }
      }
      n214 = Quotient & Remainder(x=w430, y=w429) -> (floor(x/y)=w432:u32)  [unwired: 1 out]
      n215 = Quotient & Remainder(x=w431, y=w429) -> (floor(x/y)=w428:u32)  [unwired: 1 out]
      n216 = local read "Scan rate (Hz)"() -> (w490:u32)
      n217 = call-poly <vilib>:"DAQmx Create Virtual Channel.vi"("physical channels"=w399) -> ("task out"=w472:refnum<k21>, "error out"=w471:errorcluster)  [unwired: 8 in, 5 out]
      n218 = And(x=w377, y=w378) -> (x .and. y?=w371:bool)
      n219 = And(x=w367, y=w366) -> (x .and. y?=w365:bool)
      n220 = And(x=w360, y=w361) -> (x .and. y?=w359:bool)
      n221 = And(x=w358, y=w357) -> (x .and. y?=w356:bool)
      n222 = local read "SEM Y coil"() -> (w398:tag)
      n223 = Initialize Array(i16 0 ("element"), w432, w428) -> (w355:i16[][])
      n224 = Initialize Array(i16 0 ("element"), w429, w428) -> (w354:i16[][])
      n225 = Initialize Array(i16 0 ("element"), w375, w375) -> (w350:i16[][])
      n226 = local read "X min set"() -> (w389:dbl)
      n227 = local read "X max set"() -> (w388:dbl)
      n228 = local read "X resolution"() -> (w454:u32)
      n229 = local read "Frame line rampdown ratio"() -> (w480:dbl)
      n230 = local read "Y resolution"() -> (w497:u32)
      n231 = local read "Detector B"() -> (w396:bool)
      n232 = local read "Detector D"() -> (w394:bool)
      n233 = call-poly <vilib>:"DAQmx Create Virtual Channel.vi"("task in"=w472, "physical channels"=w398, "error in"=w471) -> ("task out"=w502:refnum<k21>, "error out"=w501:errorcluster)  [unwired: 6 in, 5 out]
      n234 = case shown="True" w396 {
        tunnel: [w1577 w1585] -> w449
        tunnel: [w1578 w1584] -> w450
        tunnel: w452 -> [w1578 w1583]
        tunnel: w451 -> [w1577 w1582]
        tunnel: w385 -> [_ w1580]
        tunnel: w384 -> [_ w1579]
        frame False {
        }
        frame True {
          n235 = local read "Det B I/O"() -> (w1581:tag)
          n236 = call-poly <vilib>:"DAQmx Create Virtual Channel.vi"("task in"=w1583, "maximum value"=w1579, "minimum value"=w1580, "physical channels"=w1581, "error in"=w1582) -> ("task out"=w1584:refnum<k21>, "error out"=w1585:errorcluster)  [unwired: 4 in, 5 out]
        }
      }
      n237 = case shown="True" w395 {
        tunnel: w450 -> [w1569 w1576]
        tunnel: w449 -> [w1568 w1575]
        tunnel: [w1569 w1574] -> w448
        tunnel: [w1568 w1573] -> w447
        tunnel: w383 -> [w1566 w1570]
        tunnel: w382 -> [w1567 w1571]
        tunnel: [w1567 w1571] -> w381
        tunnel: [w1566 w1570] -> w380
        frame False {
        }
        frame True {
          n238 = local read "Det C I/O"() -> (w1572:tag)
          n239 = call-poly <vilib>:"DAQmx Create Virtual Channel.vi"("task in"=w1576, "maximum value"=w1570, "minimum value"=w1571, "physical channels"=w1572, "error in"=w1575) -> ("task out"=w1574:refnum<k21>, "error out"=w1573:errorcluster)  [unwired: 4 in, 5 out]
        }
      }
      n240 = case shown="True" w394 {
        tunnel: w448 -> [w1558 w1565]
        tunnel: w447 -> [w1557 w1564]
        tunnel: [w1558 w1563] -> w403
        tunnel: [w1557 w1562] -> w446
        tunnel: w381 -> [_ w1560]
        tunnel: w380 -> [_ w1559]
        frame False {
        }
        frame True {
          n241 = local read "Det D I/O"() -> (w1561:tag)
          n242 = call-poly <vilib>:"DAQmx Create Virtual Channel.vi"("task in"=w1565, "maximum value"=w1559, "minimum value"=w1560, "physical channels"=w1561, "error in"=w1564) -> ("task out"=w1563:refnum<k21>, "error out"=w1562:errorcluster)  [unwired: 4 in, 5 out]
        }
      }
      n243 = Multiply(x=w393, y=w490) -> (x*y=w455:u32)
      n244 = case shown="False" w371 {
        tunnel: w355 -> [_ w545]
        tunnel: [w543 w545] -> w374
        tunnel: w354 -> [_ w544]
        tunnel: [w543 w544] -> w373
        tunnel: [w543 w544] -> w372
        tunnel: w350 -> [w543 _]
        frame False {
        }
        frame True {
        }
      }
      n245 = case shown="True" w365 {
        tunnel: w355 -> [_ w542]
        tunnel: [w540 w542] -> w368
        tunnel: w354 -> [_ w541]
        tunnel: [w540 w541] -> w369
        tunnel: [w540 w541] -> w370
        tunnel: w350 -> [w540 _]
        frame False {
        }
        frame True {
        }
      }
      n246 = case shown="True" w359 {
        tunnel: w355 -> [_ w539]
        tunnel: [w537 w539] -> w364
        tunnel: w354 -> [_ w538]
        tunnel: [w537 w538] -> w363
        tunnel: [w537 w538] -> w362
        tunnel: w350 -> [w537 _]
        frame False {
        }
        frame True {
        }
      }
      n247 = case shown="True" w356 {
        tunnel: w355 -> [_ w536]
        tunnel: [w534 w536] -> w352
        tunnel: w354 -> [_ w535]
        tunnel: [w534 w535] -> w353
        tunnel: [w534 w535] -> w351
        tunnel: w350 -> [w534 _]
        frame False {
        }
        frame True {
        }
      }
      n248 = local read "AO SampClk.MaxRate"() -> (w340:dbl)
      n249 = Obtain Queue(element data type=i16[] [] ("2D array")) -> (queue out=w438:refnum<queue>, error out=w437:errorcluster)  [unwired: 3 in, 2 out]
      n250 = call "Raster line.vi"("Ramp down ratio"=w480, "Points"=w454, "End"=w388, "Start"=w389) -> ("Total points"=w379:u32, "Scan Pattern"=w482:dbl[])  [unwired: 5 in, 1 out]
      n251 = Multiply(x=w379, y=w497) -> (x*y=w496:u32)
      n252 = local read "Read AI delay (samples)"() -> (w391:i16)
      n253 = local read "Detector number"() -> (w441:u8)
      n254 = local read "Y resolution"() -> (w445:u32)
      n255 = call-poly <vilib>:"DAQmx Timing.vi"("task/channels in"=w403, "sample mode"=w487, "rate"=w455, "error in"=w446) -> ("task out"=w408:refnum<k21>, "error out"=w407:errorcluster)  [unwired: 3 in, 7 out]
      n256 = property class="DAQmx Timing"(reference=w408, error in=w407) -> (reference out=w347:refnum<k21>, error out=w349:errorcluster, "SampClk.Rate"=w469:dbl)
      n257 = Divide(x=w469, y=w393) -> (x/y=w470:dbl)
      n258 = call-poly <vilib>:"DAQmx Timing.vi"("task/channels in"=w502, "sample mode"=w500, "samples per channel"=w496, "rate"=w470, "error in"=w501) -> ("task out"=w341:refnum<k21>, "error out"=w344:errorcluster)  [unwired: 2 in, 7 out]
      n259 = call <vilib>:"DAQmx Configure Output Buffer.vi"("task/channels in"=w341, "buffer size (in samples per channel)"=w340, "error in"=w344) -> ("task out"=w342:refnum<k21>, "error out"=w343:errorcluster)  [unwired: 11 in]
      n260 = call "Get Terminal Name with Device Prefix.vi"("error in"=w343, "Local Terminal Name"="ao/StartTrigger", "task/channels in"=w342) -> ("error out"=w456:errorcluster, "Terminal Name with Device Prefix"=w457:tag, "task out"=w459:refnum<k21>)  [unwired: 6 out]
      n261 = property class="DAQmx Timing"(reference=w459, error in=w456) -> (reference out=w495:refnum<k21>, error out=w494:errorcluster, "SampClk.Rate"=w392:dbl)
      n262 = local read "AI SampClk.MaxRate"() -> (w345:dbl)
      n263 = To Long Integer(number=w445) -> (32bit integer=w444:i32)
      n264 = Multiply(x=w393, y=w379) -> (x*y=w439:u32)
      n265 = To Long Integer(number=w391) -> (32bit integer=w442:i32)
      n266 = To Long Integer(number=w441) -> (32bit integer=w443:i32)
      n267 = local read "Y min set"() -> (w386:dbl)
      n268 = local read "Y max set"() -> (w387:dbl)
      n269 = local read "Y resolution"() -> (w453:u32)
      n270 = local read "AO multiline"() -> (w413:u32)
      n271 = Multiply(x=w442, y=w443) -> (x*y=w412:i32)
      n272 = local write "AO rate"(w392) -> ()
      n273 = call <vilib>:"DAQmx Configure Input Buffer.vi"("task/channels in"=w347, "buffer size (in samples per channel)"=w345, "error in"=w349) -> ("task out"=w346:refnum<k21>, "error out"=w348:errorcluster)  [unwired: 11 in]
      n274 = property class="DAQmx Write"(reference=w495, error in=w494, "RegenMode"=w499) -> (reference out=w498:refnum<k21>, error out=w400:errorcluster)
      n275 = call "Raster line.vi"("Ramp down ratio"=0.0, "Points"=w453, "End"=w387, "Start"=w386) -> ("Scan Pattern"=w481:dbl[])  [unwired: 5 in, 2 out]
      n276 = call-poly <vilib>:"DAQmx Trigger.vi"("task/channels in"=w346, "source"=w457, "edge"=w489, "error in"=w348) -> ("task out"=w484:refnum<k21>, "error out"=w488:errorcluster)  [unwired: 10 out]
      n277 = Multiply(x=w413, y=w439) -> (x*y=w440:u32)
      n278 = call <vilib>:"DAQmx Start Task.vi"("task/channels in"=w484, "error in"=w488) -> ("task out"=w411:refnum<k21>, "error out"=w401:errorcluster)  [unwired: 12 out]
      n279 = Merge Errors(w400, w401) -> (w402:errorcluster)
      n280 = call-poly <vilib>:"DAQmx Read.vi"("task/channels in"=w411, "number of samples per channel"=w412, "error in"=w401) -> ("task out"=w410:refnum<k21>, "error out"=w409:errorcluster)  [unwired: 11 out]
      n281 = Obtain Queue(element data type=i16[] [] ("2D array")) -> (queue out=w427:refnum<queue>, error out=w493:errorcluster)  [unwired: 3 in, 2 out]
      n282 = while {
        tunnel: w438 -> [w636]
        tunnel: w437 -> [w635]
        tunnel: [w634] -> w418
        tunnel: [w633] -> w417
        shift-right: [w605] -> _
        shift-left: w373 -> [w632]
        shift-right: [w631] -> _
        shift-left: w374 -> [w606]
        shift-right: [w624] -> _
        shift-left: w369 -> [w603]
        shift-right: [w604] -> _
        shift-left: w368 -> [w618]
        shift-right: [w628] -> _
        shift-left: 0 -> [w607]
        tunnel: [w629] -> w425
        tunnel: [w627] -> w419
        tunnel: w372 -> [w625]
        tunnel: w370 -> [w623]
        shift-right: [w602] -> _
        shift-left: w364 -> [w617]
        shift-right: [w601] -> _
        shift-left: w363 -> [w622]
        tunnel: w362 -> [w621]
        shift-right: [w600] -> _
        shift-left: w352 -> [w616]
        shift-right: [w599] -> _
        shift-left: w353 -> [w620]
        tunnel: w351 -> [w619]
        tunnel: w427 -> [w615]
        tunnel: [w614] -> w426
        tunnel: w413 -> [w608]
        tunnel: [w597] -> w339
        i -> [w626]
        stop <- w597 stop-if-true
        n283 = Dequeue Element(queue=w615) -> (queue out=w614:refnum<queue>, element=w610:i16[], error out=w629:errorcluster)  [unwired: 1 in, 2 out]
        n284 = Multiply(x=w608, y=w626) -> (x*y=w609:u32)
        n285 = Array Size(array=w610) -> (size(s)=w612:i32)
        n286 = Quotient & Remainder(x=w612, y=w608) -> (floor(x/y)=w613:u32)  [unwired: 1 out]
        n287 = Reshape Array(w610, w608, w613) -> (w611:i16[][])
        n288 = for {
          tunnel: w636 -> [w733]
          tunnel: w635 -> [w732]
          tunnel: [w731] -> w634
          tunnel: [w730] -> w633
          tunnel: [w715] -> w630
          tunnel: w611 -> [w713] mode=indexing
          tunnel: w609 -> [w695]
          tunnel: w625 -> [w694]
          tunnel: w623 -> [w692]
          tunnel: w621 -> [w670]
          tunnel: w619 -> [w667]
          shift-right: [w643] -> w628
          shift-left: w607 -> [w664]
          shift-right: [w721] -> w631
          shift-left: w606 -> [w644]
          shift-right: [w663] -> w605
          shift-left: w632 -> [w722]
          shift-right: [w662] -> w604
          shift-left: w618 -> [w645]
          shift-right: [w693] -> w624
          shift-left: w603 -> [w661]
          shift-right: [w660] -> w602
          shift-left: w617 -> [w646]
          shift-right: [w659] -> w601
          shift-left: w622 -> [w671]
          shift-right: [w658] -> w600
          shift-left: w616 -> [w647]
          shift-right: [w657] -> w599
          shift-left: w620 -> [w668]
          i -> [w665]
          n289 = Add(x=w665, y=w695) -> (x+y=w666:u32)
          n290 = local read "Oversampling"() -> (w724:u16)
          n291 = local read "X resolution"() -> (w723:u32)
          n292 = local read "Detector A"() -> (w706:bool)
          n293 = local read "Detector C"() -> (w691:bool)
          n294 = local read "Detector D"() -> (w690:bool)
          n295 = local read "Detector B"() -> (w707:bool)
          n296 = Build Array(w706, w707, w691, w690) -> (w708:bool[])
          n297 = To Long Integer(number=w723) -> (32bit integer=w678:i32)
          n298 = To Long Integer(number=w724) -> (32bit integer=w681:i32)
          n299 = Boolean Array To Number(Boolean array=w708) -> (number=w705:u32)
          n300 = case shown="1, Default" w705 {
            tunnel: [w835 _ w839 _ w842 _ w849 _ w853 _ w860 _ w867 _ w876] -> w714
            tunnel: w713 -> [w835 w836 w838 w840 w843 w844 w850 w851 w854 w857 w861 w864 w868 w872 w877]
            tunnel: [_ w836 w837 _ _ w846 w848 _ _ w856 w859 _ _ w871 w875] -> w709
            tunnel: [_ _ _ w840 w841 w845 w847 _ _ _ _ w863 w866 w869 w874] -> w680
            tunnel: [_ _ _ _ _ _ _ w851 w852 w855 w858 w862 w865 w870 w873] -> w679
            frame 1, Default {
            }
            frame 2 {
            }
            frame 3 {
              n301 = Decimate 1D Array(w838) -> (w839:i16[], w837:i16[])
            }
            frame 4 {
            }
            frame 5 {
              n302 = Decimate 1D Array(w843) -> (w842:i16[], w841:i16[])
            }
            frame 6 {
              n303 = Decimate 1D Array(w844) -> (w846:i16[], w845:i16[])
            }
            frame 7 {
              n304 = Decimate 1D Array(w850) -> (w849:i16[], w848:i16[], w847:i16[])
            }
            frame 8 {
            }
            frame 9 {
              n305 = Decimate 1D Array(w854) -> (w853:i16[], w852:i16[])
            }
            frame 10 {
              n306 = Decimate 1D Array(w857) -> (w856:i16[], w855:i16[])
            }
            frame 11 {
              n307 = Decimate 1D Array(w861) -> (w860:i16[], w859:i16[], w858:i16[])
            }
            frame 12 {
              n308 = Decimate 1D Array(w864) -> (w863:i16[], w862:i16[])
            }
            frame 13 {
              n309 = Decimate 1D Array(w868) -> (w867:i16[], w866:i16[], w865:i16[])
            }
            frame 14 {
              n310 = Decimate 1D Array(w872) -> (w871:i16[], w869:i16[], w870:i16[])
            }
            frame 15 {
              n311 = Decimate 1D Array(w877) -> (w876:i16[], w875:i16[], w874:i16[], w873:i16[])
            }
          }
          n312 = local read "Decimating factor"() -> (w720:u16)
          n313 = To Double Precision Float(number=w714) -> (double precision float=w704:dbl[])
          n314 = To Double Precision Float(number=w709) -> (double precision float=w703:dbl[])
          n315 = To Double Precision Float(number=w680) -> (double precision float=w688:dbl[])
          n316 = To Double Precision Float(number=w679) -> (double precision float=w689:dbl[])
          n317 = To Long Integer(number=w720) -> (32bit integer=w672:i32)
          n318 = call-poly <vilib>:"Decimate (single shot).vi"("averaging"=TRUE, "decimating factor"=w681, "X"=w704) -> ("Decimated Array"=w719:dbl[])  [unwired: 8 out]
          n319 = call-poly <vilib>:"Decimate (single shot).vi"("averaging"=TRUE, "decimating factor"=w681, "X"=w703) -> ("Decimated Array"=w725:dbl[])  [unwired: 8 out]
          n320 = call-poly <vilib>:"Decimate (single shot).vi"("averaging"=TRUE, "decimating factor"=w681, "X"=w688) -> ("Decimated Array"=w687:dbl[])  [unwired: 8 out]
          n321 = call-poly <vilib>:"Decimate (single shot).vi"("averaging"=TRUE, "decimating factor"=w681, "X"=w689) -> ("Decimated Array"=w686:dbl[])  [unwired: 8 out]
          n322 = Quotient & Remainder(x=w666, y=w672) -> (x-y*floor(x/y)=w641:u32, floor(x/y)=w673:u32)
          n323 = Increment(x=w641) -> (x+1=w642:u32)
          n324 = To Word Integer(number=w719) -> (16bit integer=w729:i16[])
          n325 = To Word Integer(number=w725) -> (16bit integer=w726:i16[])
          n326 = To Word Integer(number=w687) -> (16bit integer=w682:i16[])
          n327 = To Word Integer(number=w686) -> (16bit integer=w685:i16[])
          n328 = Equal?(x=w642, y=w672) -> (x = y?=w669:bool)
          n329 = Array Subset(array=w729, length=w678) -> (w712:i16[])  [unwired: 1 in]
          n330 = Array Subset(array=w726, length=w678) -> (w711:i16[])  [unwired: 1 in]
          n331 = Array Subset(array=w682, length=w678) -> (w676:i16[])  [unwired: 1 in]
          n332 = Array Subset(array=w685, length=w678) -> (w675:i16[])  [unwired: 1 in]
          n333 = local read "Detector A"() -> (w656:bool)
          n334 = local read "Display"() -> (w648:bool)
          n335 = local read "Detector B"() -> (w654:bool)
          n336 = local read "Detector C"() -> (w651:bool)
          n337 = local read "Detector D"() -> (w649:bool)
          n338 = case shown="4" w705 {
            tunnel: w712 -> [w792 _ w796 _ w799 _ w807 _ w811 _ w818 _ w825 _ w834]
            tunnel: w711 -> [_ w793 w795 _ _ w803 w806 _ _ w814 w817 _ _ w829 w833]
            tunnel: [w792 w793 w794 w797 w800 w801 w804 w808 w809 w812 w815 w819 w822 w826 w830] -> w710
            tunnel: w676 -> [_ _ _ w797 w798 w802 w805 _ _ _ _ w820 w824 w828 w832]
            tunnel: w675 -> [_ _ _ _ _ _ _ w808 w810 w813 w816 w821 w823 w827 w831]
            frame 1, Default {
            }
            frame 2 {
            }
            frame 3 {
              n339 = Interleave 1D Arrays(w796, w795) -> (w794:i16[])
            }
            frame 4 {
            }
            frame 5 {
              n340 = Interleave 1D Arrays(w799, w798) -> (w800:i16[])
            }
            frame 6 {
              n341 = Interleave 1D Arrays(w803, w802) -> (w801:i16[])
            }
            frame 7 {
              n342 = Interleave 1D Arrays(w807, w806, w805) -> (w804:i16[])
            }
            frame 8 {
            }
            frame 9 {
              n343 = Interleave 1D Arrays(w811, w810) -> (w809:i16[])
            }
            frame 10 {
              n344 = Interleave 1D Arrays(w814, w813) -> (w812:i16[])
            }
            frame 11 {
              n345 = Interleave 1D Arrays(w818, w817, w816) -> (w815:i16[])
            }
            frame 12 {
              n346 = Interleave 1D Arrays(w820, w821) -> (w819:i16[])
            }
            frame 13 {
              n347 = Interleave 1D Arrays(w825, w824, w823) -> (w822:i16[])
            }
            frame 14 {
              n348 = Interleave 1D Arrays(w829, w828, w827) -> (w826:i16[])
            }
            frame 15 {
              n349 = Interleave 1D Arrays(w834, w833, w832, w831) -> (w830:i16[])
            }
          }
          n350 = To Double Precision Float(number=w712) -> (double precision float=w696:dbl[])
          n351 = To Double Precision Float(number=w711) -> (double precision float=w697:dbl[])
          n352 = To Double Precision Float(number=w676) -> (double precision float=w677:dbl[])
          n353 = To Double Precision Float(number=w675) -> (double precision float=w674:dbl[])
          n354 = And(x=w656, y=w648) -> (x .and. y?=w655:bool)
          n355 = And(x=w648, y=w654) -> (x .and. y?=w653:bool)
          n356 = And(x=w648, y=w651) -> (x .and. y?=w652:bool)
          n357 = And(x=w648, y=w649) -> (x .and. y?=w650:bool)
          n358 = local read "Save"() -> (w638:bool)
          n359 = local read "Detector number"() -> (w700:u8)
          n360 = case shown="True" w655 {
            tunnel: w696 -> [_ w920]
            tunnel: w722 -> [w907 w915]
            tunnel: [w908 w923] -> w721
            tunnel: w644 -> [w908 w922]
            tunnel: w672 -> [_ w918]
            tunnel: [w907 w921] -> w663
            tunnel: w641 -> [_ w914]
            tunnel: w694 -> [_ w913]
            tunnel: w669 -> [_ w909]
            tunnel: w673 -> [_ w910]
            frame False {
            }
            frame True {
              n361 = call-poly <vilib>:"Decimate (single shot).vi"("averaging"=TRUE, "decimating factor"=w918, "X"=w920) -> ("Decimated Array"=w912:dbl[])  [unwired: 8 out]
              n362 = To Word Integer(number=w912) -> (16bit integer=w916:i16[])
              n363 = Replace Array Subset(array=w915, new element=w916, index (row)=w914) -> (w917:i16[][])  [unwired: 1 in]
              n364 = Array Size(array=w912) -> (size(s)=w911:i32)
              n365 = case shown="True" w909 {
                tunnel: [w925 w926] -> w923
                tunnel: w922 -> [w925 w928]
                tunnel: w918 -> [_ w935]
                tunnel: [w924 w933] -> w921
                tunnel: w917 -> [w924 w934]
                tunnel: w913 -> [_ w933]
                tunnel: w911 -> [_ w929]
                tunnel: w910 -> [_ w927]
                frame False {
                }
                frame True {
                  n366 = call "2D Array Decimate.vi"("y decimating factor"=w935, "Input 2D Array"=w934) -> ("output array"=w930:dbl[][])  [unwired: 2 in, 7 out]
                  n367 = To Word Integer(number=w930) -> (16bit integer=w931:i16[][])
                  n368 = Reshape Array(w931, w929) -> (w932:i16[])
                  n369 = Replace Array Subset(array=w928, new element=w932, index (row)=w927) -> (w926:i16[][])  [unwired: 1 in]
                  "Det A Img" <- w926
                  n370 = shared-variable ".\\Zeiss Library.lvlib\\Det A Img"(w926) -> ()  [unwired: 2 out]
                }
              }
            }
          }
          n371 = case shown="True" w653 {
            tunnel: w672 -> [_ w890]
            tunnel: w697 -> [_ w891]
            tunnel: w661 -> [w878 w882]
            tunnel: [w879 w894] -> w662
            tunnel: w645 -> [w879 w893]
            tunnel: w669 -> [_ w889]
            tunnel: w673 -> [_ w888]
            tunnel: w641 -> [_ w886]
            tunnel: [w878 w881] -> w693
            tunnel: w692 -> [_ w880]
            frame False {
            }
            frame True {
              n372 = call-poly <vilib>:"Decimate (single shot).vi"("averaging"=TRUE, "decimating factor"=w890, "X"=w891) -> ("Decimated Array"=w885:dbl[])  [unwired: 8 out]
              n373 = To Word Integer(number=w885) -> (16bit integer=w887:i16[])
              n374 = Replace Array Subset(array=w882, new element=w887, index (row)=w886) -> (w884:i16[][])  [unwired: 1 in]
              n375 = Array Size(array=w885) -> (size(s)=w883:i32)
              n376 = case shown="True" w889 {
                tunnel: w890 -> [_ w906]
                tunnel: [w896 w897] -> w894
                tunnel: w893 -> [w896 w904]
                tunnel: w888 -> [_ w903]
                tunnel: w884 -> [w895 w899]
                tunnel: w883 -> [_ w900]
                tunnel: [w895 w898] -> w881
                tunnel: w880 -> [_ w898]
                frame False {
                }
                frame True {
                  n377 = call "2D Array Decimate.vi"("y decimating factor"=w906, "Input 2D Array"=w899) -> ("output array"=w905:dbl[][])  [unwired: 2 in, 7 out]
                  n378 = To Word Integer(number=w905) -> (16bit integer=w901:i16[][])
                  n379 = Reshape Array(w901, w900) -> (w902:i16[])
                  n380 = Replace Array Subset(array=w904, new element=w902, index (row)=w903) -> (w897:i16[][])  [unwired: 1 in]
                  "Det B Img" <- w897
                  n381 = shared-variable ".\\Zeiss Library.lvlib\\Det B Img"(w897) -> ()  [unwired: 2 out]
                }
              }
            }
          }
          n382 = case shown="True" w652 {
            tunnel: w672 -> [_ w775]
            tunnel: w677 -> [_ w776]
            tunnel: w671 -> [w763 w767]
            tunnel: [w764 w779] -> w660
            tunnel: w646 -> [w764 w778]
            tunnel: w669 -> [_ w774]
            tunnel: w673 -> [_ w773]
            tunnel: w641 -> [_ w771]
            tunnel: [w763 w766] -> w659
            tunnel: w670 -> [_ w765]
            frame False {
            }
            frame True {
              n383 = call-poly <vilib>:"Decimate (single shot).vi"("averaging"=TRUE, "decimating factor"=w775, "X"=w776) -> ("Decimated Array"=w770:dbl[])  [unwired: 8 out]
              n384 = To Word Integer(number=w770) -> (16bit integer=w772:i16[])
              n385 = Replace Array Subset(array=w767, new element=w772, index (row)=w771) -> (w769:i16[][])  [unwired: 1 in]
              n386 = Array Size(array=w770) -> (size(s)=w768:i32)
              n387 = case shown="True" w774 {
                tunnel: w775 -> [_ w791]
                tunnel: [w781 w782] -> w779
                tunnel: w778 -> [w781 w789]
                tunnel: w773 -> [_ w788]
                tunnel: w769 -> [w780 w784]
                tunnel: w768 -> [_ w785]
                tunnel: [w780 w783] -> w766
                tunnel: w765 -> [_ w783]
                frame False {
                }
                frame True {
                  n388 = call "2D Array Decimate.vi"("y decimating factor"=w791, "Input 2D Array"=w784) -> ("output array"=w790:dbl[][])  [unwired: 2 in, 7 out]
                  n389 = To Word Integer(number=w790) -> (16bit integer=w786:i16[][])
                  n390 = Reshape Array(w786, w785) -> (w787:i16[])
                  n391 = Replace Array Subset(array=w789, new element=w787, index (row)=w788) -> (w782:i16[][])  [unwired: 1 in]
                  "Det C Img" <- w782
                  n392 = shared-variable ".\\Zeiss Library.lvlib\\Det C Img"(w782) -> ()  [unwired: 2 out]
                }
              }
            }
          }
          n393 = case shown="True" w650 {
            tunnel: w672 -> [_ w746]
            tunnel: w674 -> [_ w747]
            tunnel: w668 -> [w734 w738]
            tunnel: [w735 w750] -> w658
            tunnel: w647 -> [w735 w749]
            tunnel: w669 -> [_ w745]
            tunnel: w673 -> [_ w744]
            tunnel: w641 -> [_ w742]
            tunnel: [w734 w737] -> w657
            tunnel: w667 -> [_ w736]
            frame False {
            }
            frame True {
              n394 = call-poly <vilib>:"Decimate (single shot).vi"("averaging"=TRUE, "decimating factor"=w746, "X"=w747) -> ("Decimated Array"=w741:dbl[])  [unwired: 8 out]
              n395 = To Word Integer(number=w741) -> (16bit integer=w743:i16[])
              n396 = Replace Array Subset(array=w738, new element=w743, index (row)=w742) -> (w740:i16[][])  [unwired: 1 in]
              n397 = Array Size(array=w741) -> (size(s)=w739:i32)
              n398 = case shown="True" w745 {
                tunnel: w746 -> [_ w762]
                tunnel: [w752 w753] -> w750
                tunnel: w749 -> [w752 w760]
                tunnel: w744 -> [_ w759]
                tunnel: w740 -> [w751 w755]
                tunnel: w739 -> [_ w756]
                tunnel: [w751 w754] -> w737
                tunnel: w736 -> [_ w754]
                frame False {
                }
                frame True {
                  n399 = call "2D Array Decimate.vi"("y decimating factor"=w762, "Input 2D Array"=w755) -> ("output array"=w761:dbl[][])  [unwired: 2 in, 7 out]
                  n400 = To Word Integer(number=w761) -> (16bit integer=w757:i16[][])
                  n401 = Reshape Array(w757, w756) -> (w758:i16[])
                  n402 = Replace Array Subset(array=w760, new element=w758, index (row)=w759) -> (w753:i16[][])  [unwired: 1 in]
                  "Det D Img" <- w753
                  n403 = shared-variable ".\\Zeiss Library.lvlib\\Det D Img"(w753) -> ()  [unwired: 2 out]
                }
              }
            }
          }
          n404 = Array Size(array=w710) -> (size(s)=w701:i32)
          n405 = local read "PNG only"() -> (w640:bool)
          n406 = Not(x=w640) -> (.not. x?=w639:bool)
          n407 = To Long Integer(number=w700) -> (32bit integer=w699:i32)
          n408 = And(x=w638, y=w639) -> (x .and. y?=w637:bool)
          n409 = Quotient & Remainder(x=w701, y=w699) -> (floor(x/y)=w702:i32)  [unwired: 1 out]
          n410 = Add(x=w702, y=w664) -> (x+y=w643:i32)
          n411 = case shown="True" w637 {
            tunnel: w733 -> [w937 w942]
            tunnel: w732 -> [w936 w941]
            tunnel: [w937 w940] -> w731
            tunnel: [w936 w939] -> w730
            tunnel: w710 -> [_ w938]
            frame False {
            }
            frame True {
              n412 = Enqueue Element(queue=w942, element=w938, error in (no error)=w941) -> (queue out=w940:refnum<queue>, error out=w939:errorcluster)  [unwired: 2 out]
            }
          }
          n413 = local write "Total pixels recorded"(w643) -> ()
          n414 = local read "X resolution"() -> (w718:u32)
          n415 = local read "Y resolution"() -> (w717:u32)
          n416 = Multiply(x=w718, y=w717) -> (x*y=w716:u32)
          n417 = To Unsigned Long Integer(number=w643) -> (unsigned 32bit integer=w698:u32)
          n418 = Greater Or Equal?(x=w698, y=w716) -> (x >= y?=w715:bool)
        }
        n419 = Unbundle By Name(w629) -> ("status"=w627:bool)
        n420 = local read "stop"() -> (w598:bool)
        n421 = Compound Arithmetic op=OR(w630, w627, w598) -> (w597:bool)
      }
      n422 = while {
        tunnel: w498 -> [w574]
        tunnel: w402 -> [w573]
        tunnel: [w572] -> w337
        tunnel: [w571] -> w478
        tunnel: w482 -> [w560]
        tunnel: w481 -> [w559]
        tunnel: w413 -> [w553]
        tunnel: w379 -> [w546]
        i -> [w568]
        stop <- w575 stop-if-true
        n423 = To Long Integer(number=w553) -> (32bit integer=w557:i32)
        n424 = Increment(x=w568) -> (x+1=w561:i32)
        n425 = To Long Integer(number=w553) -> (32bit integer=w556:i32)
        n426 = local read "Y resolution"() -> (w570:u32)
        n427 = Multiply(x=w557, y=w568) -> (x*y=w567:i32)
        n428 = To Unsigned Long Integer(number=w561) -> (unsigned 32bit integer=w555:u32)
        n429 = Array Subset(array=w559, index=w567, length=w556) -> (w566:dbl[])
        n430 = Multiply(x=w553, y=w555) -> (x*y=w552:u32)
        n431 = Less Or Equal?(x=w570, y=w552) -> (x <= y?=w576:bool)
        n432 = local write "AO scan line"(w552) -> ()
        n433 = for {
          N: w553 -> [_]
          tunnel: [w582] -> _ mode=indexing
          tunnel: w560 -> [w582]
          tunnel: [w582] -> w569 mode=indexing
          tunnel: w566 -> [w581] mode=indexing
          tunnel: [w580] -> w565 mode=indexing
          tunnel: w546 -> [w579]
          n434 = Initialize Array(w581, w579) -> (w580:dbl[])
        }
        n435 = Multiply(x=w553, y=w546) -> (x*y=w564:u32)
        n436 = To Long Integer(number=w564) -> (32bit integer=w554:i32)
        n437 = Reshape Array(w569, w554) -> (w558:dbl[])
        n438 = Reshape Array(w565, w554) -> (w563:dbl[])
        n439 = local read "stop"() -> (w547:bool)
        n440 = Build Array(w558, w563) -> (w562:dbl[][])
        n441 = call-poly <vilib>:"DAQmx Write.vi"("task/channels in"=w574, "auto start"=TRUE, "data"=w562, "error in"=w573) -> ("task out"=w572:refnum<k21>, "error out"=w571:errorcluster)  [unwired: 10 out]
        n442 = Array Max & Min(array=w558) -> (max value=w548:dbl, max index (indices)=w549:i32, min value=w550:dbl, min index (indices)=w551:i32)
        n443 = local write "X min (V)"(w550) -> ()
        n444 = local write "X max (V)"(w548) -> ()
        n445 = Unbundle By Name(w571) -> ("status"=w577:bool)
        n446 = Compound Arithmetic op=OR(w577, w576, w547) -> (w575:bool)
        n447 = local write "X min index"(w551) -> ()
        n448 = local write "X max index"(w549) -> ()
      }
      n449 = while {
        tunnel: w409 -> [w1610]
        tunnel: [w1624] -> w406
        tunnel: [w1623] -> w405
        tunnel: w410 -> [w1611]
        tunnel: w440 -> [w1617]
        tunnel: w427 -> [w1626]
        tunnel: w493 -> [w1625]
        tunnel: [w1620] -> w468
        tunnel: [w1619] -> w465
        tunnel: [w1618] -> w461
        tunnel: w444 -> [w1614]
        tunnel: w413 -> [w1612]
        tunnel: [w1609] -> w335
        i -> [w1615]
        stop <- w1609 stop-if-true
        n450 = property class="DAQmx Read"(reference=w1611, error in=w1610) -> (reference out=w1621:refnum<k21>, error out=w1622:errorcluster, "AvailSampPerChan"=w1608:u32)
        n451 = Increment(x=w1615) -> (x+1=w1613:i32)
        n452 = Multiply(x=w1612, y=w1613) -> (x*y=w1607:u32)
        n453 = local write "AvailSampPerChan"(w1608) -> ()
        n454 = local write "Total lines scanned"(w1607) -> ()
        n455 = call-poly <vilib>:"DAQmx Read.vi"("task/channels in"=w1621, "number of samples per channel"=w1617, "error in"=w1622) -> ("task out"=w1624:refnum<k21>, "data"=w1616:i16[], "error out"=w1623:errorcluster)  [unwired: 10 out]
        n456 = Greater Or Equal?(x=w1607, y=w1614) -> (x >= y?=w1627:bool)
        n457 = Enqueue Element(queue=w1626, element=w1616, error in (no error)=w1625) -> (queue out=w1620:refnum<queue>, error out=w1619:errorcluster)  [unwired: 2 out]
        n458 = Unbundle By Name(w1623) -> ("status"=w1618:bool)
        n459 = local read "stop"() -> (w1606:bool)
        n460 = Compound Arithmetic op=OR(w1618, w1627, w1606) -> (w1609:bool)
      }
      n461 = while {
        tunnel: w406 -> [w590]
        tunnel: [w590] -> w336
        tunnel: [w589] -> w404
        tunnel: w405 -> [w589]
        stop <- w586 stop-if-true
        n462 = local read "Header done?"() -> (w583:bool)
        n463 = local read "Save"() -> (w587:bool)
        n464 = local read "stop"() -> (w584:bool)
        n465 = Not(x=w587) -> (.not. x?=w585:bool)
        n466 = Wait Until Next ms Multiple(millisecond multiple=u32 500 ("milliseconds to wait")) -> ()  [unwired: 1 out]
        n467 = Compound Arithmetic op=OR(w583, w585, w584) -> (w586:bool)
      }
      n468 = Get Queue Status(queue=w468, error in (no error)=w465) -> (queue out=w466:refnum<queue>, error out=w464:errorcluster, # elements in queue=w463:i32)  [unwired: 6 out]
      n469 = flat-sequence {
        tunnel: w335 -> [_]
        frame #0 {
          w525 = TRUE ("Initialization")
          w509 = T12 3 items=["no dialog", "OK message", "continue or stop message", "OK message + warnings", "continue/stop + warnings"] ("type of dialog (OK msg:1)")
          w505 = 0 items=["one channel for each line", "one channel for all lines"] ("line grouping")
          n470 = local read "COM port"() -> (w522:refnum<visa-resource-name>)
          n471 = local read "Detector FIB-NI auto switch"() -> (w513:tag)
          n472 = call "Remcon32 command.vi"("Initialization"=w525, "SEM command"="bblk 1" ("write buffer"), "COM port in"=w522) -> ("error out"=w524:errorcluster, "COM port out"=w523:refnum<visa-resource-name>)  [unwired: 2 in, 5 out]
          n473 = call-poly <vilib>:"DAQmx Create Virtual Channel.vi"("lines"=w513, "line grouping"=w505) -> ("task out"=w503:refnum<k21>, "error out"=w504:errorcluster)  [unwired: 3 in, 9 out]
          n474 = call "Remcon32 command.vi"("error in"=w524, "SEM command"="edx 0" ("write buffer"), "COM port in"=w523) -> ("error out"=w517:errorcluster, "COM port out"=w515:refnum<visa-resource-name>)  [unwired: 2 in, 5 out]
          n475 = call <vilib>:"DAQmx Start Task.vi"("task/channels in"=w503, "error in"=w504) -> ("task out"=w506:refnum<k21>, "error out"=w507:errorcluster)  [unwired: 12 out]
          n476 = call "Remcon32 command.vi"("error in"=w517, "SEM command"="bblk 1" ("write buffer"), "COM port in"=w515) -> ("error out"=w518:errorcluster, "COM port out"=w516:refnum<visa-resource-name>)  [unwired: 2 in, 5 out]
          n477 = local read "Freeze"() -> (w520:bool)
          n478 = call-poly <vilib>:"DAQmx Write.vi"("task/channels in"=w506, "data"=FALSE, "error in"=w507) -> ("task out"=w511:refnum<k21>, "error out"=w512:errorcluster)  [unwired: 1 in, 10 out]
          n479 = case shown="True" w520 {
            tunnel: w516 -> [w528 w532]
            tunnel: w525 -> [w526 w531]
            tunnel: w518 -> [w527 w530]
            frame False {
              n480 = call "Remcon32 command.vi"("Close session"=w526, "error in"=w527, "COM port in"=w528) -> ()  [unwired: 2 in, 7 out]
            }
            frame True {
              n481 = call "Remcon32 command.vi"("Close session"=w531, "error in"=w530, "SEM command"="frez" ("write buffer"), "COM port in"=w532) -> ()  [unwired: 1 in, 7 out]
            }
          }
          n482 = call <vilib>:"DAQmx Clear Task.vi"("task in"=w511, "error in"=w512) -> ("error out"=w510:errorcluster)  [unwired: 13 out]
          n483 = call <vilib>:"Simple Error Handler.vi"("type of dialog (OK msg:1)"=w509, "error in (no error)"=w510) -> ()  [unwired: 8 out]
        }
      }
      n484 = case shown="True" w335 {
        tunnel: w337 -> [w1603 w1605]
        tunnel: [w1602 w1605] -> w479
        tunnel: w478 -> [w1601 w1604]
        tunnel: [w1600 w1604] -> w475
        frame False {
          n485 = call <vilib>:"DAQmx Wait Until Done.vi"("task/channels in"=w1603, "timeout (sec)"=-1.0, "error in"=w1601) -> ("task out"=w1602:refnum<k21>, "error out"=w1600:errorcluster)  [unwired: 11 out]
        }
        frame True {
        }
      }
      n486 = Equal To 0?(x=w463) -> (x = 0?=w462:bool)
      n487 = Compound Arithmetic op=OR(w462, w461) -> (w460:bool)
      n488 = call <vilib>:"DAQmx Stop Task.vi"("task/channels in"=w336, "error in"=w404) -> ("task out"=w474:refnum<k21>, "error out"=w473:errorcluster)  [unwired: 12 out]
      n489 = case shown="True" w460 {
        tunnel: w466 -> [_ w1598]
        tunnel: w464 -> [w1595 w1597]
        tunnel: [w1595 w1596] -> w467
        frame False {
        }
        frame True {
          n490 = Release Queue(queue=w1598, error in (no error)=w1597) -> (error out=w1596:errorcluster)  [unwired: 3 out]
        }
      }
      n491 = call <vilib>:"DAQmx Stop Task.vi"("task/channels in"=w479, "error in"=w475) -> ("task out"=w477:refnum<k21>, "error out"=w476:errorcluster)  [unwired: 12 out]
      n492 = call <vilib>:"DAQmx Clear Task.vi"("task in"=w474, "error in"=w473) -> ("error out"=w485:errorcluster)  [unwired: 13 out]
      n493 = Generate Occurrence() -> (w338:refnum<k4>)
      n494 = case shown="True" w390 {
        tunnel: w438 -> [_ w947]
        tunnel: [_ w946] -> w416
        tunnel: [_ w945] -> w415
        tunnel: w403 -> [_ w944]
        tunnel: w338 -> [_ w943]
        frame False {
        }
        frame True {
          n495 = stacked-sequence {
            tunnel: w947 -> [_ _ w1030 _]
            tunnel: [_ _ w1029 _] -> w946
            tunnel: [_ _ w1028 _] -> w945
            tunnel: w944 -> [_ _ w1027 _]
            tunnel: w943 -> [_ _ w1025 _]
            frame #0 {
              n496 = local read "File path"() -> (w949:path)
              n497 = Get Date/Time In Seconds() -> (seconds since 1Jan1904=w952:timestamp)
              n498 = Get Date/Time In Seconds() -> (seconds since 1Jan1904=w958:timestamp)
              n499 = Format Date/Time String(time format string (%c)="%y-%m-%d_%H%M%S", seconds (now)=w952) -> (date/time string=w951:string)  [unwired: 1 out]
              n500 = Format Date/Time String(time format string (%c)="Y%Y\\M%m\\D%d", seconds (now)=w958) -> (date/time string=w959:string)  [unwired: 1 out]
              n501 = Concatenate Strings("Zeiss_" ("string"), w951, ".dat" ("string")) -> (w956:string)
              n502 = Build Path(base path=w949, name or relative path=w959) -> (appended path=w948:path)
              n503 = File/Directory Info(path=w948) -> (path out=w962:path, error out=w960:errorcluster)  [unwired: 1 in, 5 out]
              n504 = Build Path(base path=w948, name or relative path=w956) -> (appended path=→"File name":path)
              n505 = Unbundle By Name(w960) -> ("status"=w961:bool)
              n506 = case shown="True" w961 {
                tunnel: w962 -> [_ w963]
                frame False {
                }
                frame True {
                  n507 = Create Folder(path (use dialog)=w963) -> ()  [unwired: 1 in, 4 out]
                }
              }
            }
            frame #1 {
              n508 = local read "PNG only"() -> (w964:bool)
              n509 = case shown="False" w964 {
                frame False {
                  w993 = ".csv" ("string")
                  n510 = Get Date/Time In Seconds() -> (seconds since 1Jan1904=w991:timestamp)
                  n511 = Get Date/Time In Seconds() -> (seconds since 1Jan1904=w989:timestamp)
                  n512 = Get Date/Time In Seconds() -> (seconds since 1Jan1904=w986:timestamp)
                  n513 = local read "File path"() -> (w965:path)
                  n514 = Format Date/Time String(time format string (%c)="Y%Y\\%Y", seconds (now)=w991) -> (date/time string=w990:string)  [unwired: 1 out]
                  n515 = Format Date/Time String(time format string (%c)="Y%Y\\M%m\\%Y-%m", seconds (now)=w989) -> (date/time string=w984:string)  [unwired: 1 out]
                  n516 = Format Date/Time String(time format string (%c)="Y%Y\\M%m\\D%d\\%Y-%m-%d", seconds (now)=w986) -> (date/time string=w985:string)  [unwired: 1 out]
                  n517 = Concatenate Strings(w990, w993) -> (w983:string)
                  n518 = Concatenate Strings(w984, w993) -> (w982:string)
                  n519 = Concatenate Strings(w985, w993) -> (w981:string)
                  n520 = Build Path(base path=w965, name or relative path=w983) -> (appended path=w980:path)
                  n521 = Build Path(base path=w965, name or relative path=w982) -> (appended path=w974:path)
                  n522 = Build Path(base path=w965, name or relative path=w981) -> (appended path=w970:path)
                  n523 = File/Directory Info(path=w980) -> (path out=w979:path, error out=w994:errorcluster)  [unwired: 1 in, 5 out]
                  n524 = File/Directory Info(path=w974) -> (path out=w976:path, error out=w975:errorcluster)  [unwired: 1 in, 5 out]
                  n525 = File/Directory Info(path=w970) -> (path out=w972:path, error out=w971:errorcluster)  [unwired: 1 in, 5 out]
                  n526 = Unbundle By Name(w994) -> ("status"=w978:bool)
                  n527 = Unbundle By Name(w975) -> ("status"=w977:bool)
                  n528 = Unbundle By Name(w971) -> ("status"=w973:bool)
                  n529 = Array To Spreadsheet String(delimiter (Tab)="," ("string"), array=string[] ["Date", "Time", "Notes", "Detector A", "Detector B", "Detector C", "Detector D", "Detectors", "X resolution", "Y resolution", "Rate (Hz)", "Brightness A (%)", "Contrast A (%)", "Brightness B (%)", "Contrast B (%)", "Magnification", "Pixel size (nm)", "Working Distance (mm)", "EHT (kV)", "Aperture #", "High current mode", "Probe current (A)", "Beam shift X", "Beam shift Y", "Stigmation X", "Stigmation Y", "Alignment X", "Alignment Y", "FIB spacing (nm)", "A Img Focus Index", "B Img Focus Index", "C Img Focus Index", "D Img Focus Index"], 3:"%s" ("format string")) -> (spreadsheet string=w967:string)
                  n530 = case shown="True" w978 {
                    tunnel: w979 -> [_ w1024]
                    tunnel: w967 -> [_ w1015]
                    frame False {
                    }
                    frame True {
                      n531 = Open/Create/Replace File(file path (use dialog)=w1024, operation (0:open)=T11."create") -> (refnum out=w1022:refnum<file>, error out=w1021:errorcluster)  [unwired: 1 in, 4 out]
                      n532 = Set File Position(refnum=w1022, from (0:start)=enum16{"start", "end", "current"}."start", error in=w1021) -> (refnum out=w1020:refnum<file>, error out=w1023:errorcluster)  [unwired: 1 out]
                      n533 = Write to Text File(file (use dialog)=w1020, text=w1015, error in=w1023) -> (refnum out=w1019:refnum<file>, error out=w1018:errorcluster)  [unwired: 2 out]
                      n534 = Close File(refnum=w1019, error in=w1018) -> ()  [unwired: 2 out]
                    }
                  }
                  n535 = case shown="True" w977 {
                    tunnel: w976 -> [_ w1014]
                    tunnel: w967 -> [_ w1005]
                    frame False {
                    }
                    frame True {
                      n536 = Open/Create/Replace File(file path (use dialog)=w1014, operation (0:open)=T11."create") -> (refnum out=w1012:refnum<file>, error out=w1011:errorcluster)  [unwired: 1 in, 4 out]
                      n537 = Set File Position(refnum=w1012, from (0:start)=enum16{"start", "end", "current"}."start", error in=w1011) -> (refnum out=w1010:refnum<file>, error out=w1013:errorcluster)  [unwired: 1 out]
                      n538 = Write to Text File(file (use dialog)=w1010, text=w1005, error in=w1013) -> (refnum out=w1009:refnum<file>, error out=w1008:errorcluster)  [unwired: 2 out]
                      n539 = Close File(refnum=w1009, error in=w1008) -> ()  [unwired: 2 out]
                    }
                  }
                  n540 = case shown="True" w973 {
                    tunnel: w972 -> [_ w1004]
                    tunnel: w967 -> [_ w995]
                    frame False {
                    }
                    frame True {
                      n541 = Open/Create/Replace File(file path (use dialog)=w1004, operation (0:open)=T11."create") -> (refnum out=w1002:refnum<file>, error out=w1001:errorcluster)  [unwired: 1 in, 4 out]
                      n542 = Set File Position(refnum=w1002, from (0:start)=enum16{"start", "end", "current"}."start", error in=w1001) -> (refnum out=w1000:refnum<file>, error out=w1003:errorcluster)  [unwired: 1 out]
                      n543 = Write to Text File(file (use dialog)=w1000, text=w995, error in=w1003) -> (refnum out=w999:refnum<file>, error out=w998:errorcluster)  [unwired: 2 out]
                      n544 = Close File(refnum=w999, error in=w998) -> ()  [unwired: 2 out]
                    }
                  }
                }
                frame True {
                }
              }
            }
            frame #2 {
              n545 = local read "PNG only"() -> (w1026:bool)
              n546 = case shown="False" w1026 {
                tunnel: w1030 -> [w1098 _]
                tunnel: [w1097 _] -> w1029
                tunnel: [w1096 _] -> w1028
                tunnel: w1027 -> [w1095 _]
                tunnel: w1025 -> [_ w1347]
                frame False {
                  w1113 = "\"" ("string")
                  w1129 = ".csv" ("string")
                  w1131 = T11."open or create" ("operation (0:open)")
                  w1130 = enum16{"start", "end", "current"}."end" ("from (0:start)")
                  w1186 = T12 3 items=["no dialog", "OK message", "continue or stop message", "OK message + warnings", "continue/stop + warnings"] ("type of dialog (OK msg:1)")
                  # "Save daily runsheet"
                  # "Save yearly runsheet"
                  # "Save monthly runsheet"
                  n547 = local read "X resolution"() -> (w1127:u32)
                  n548 = local read "Y resolution"() -> (w1182:u32)
                  n549 = local read "Oversampling"() -> (w1183:u16)
                  n550 = local read "Read AI delay (samples)"() -> (w1170:i16)
                  n551 = local read "Scan speed"() -> (w1171:u8)
                  n552 = local read "AO rate"() -> (w1184:dbl)
                  n553 = local read "Frame line rampdown ratio"() -> (w1185:dbl)
                  n554 = local read "X min (V)"() -> (w1106:dbl)
                  n555 = local read "X max (V)"() -> (w1105:dbl)
                  n556 = local read "File name"() -> (w1031:path)
                  n557 = Bundle("X resolution"=w1127, "Y resolution"=w1182, "Oversampling"=w1183, "Read AI delay (samples)"=w1170, "Scan speed"=w1171, "AO rate"=w1184, "Frame line rampdown ratio"=w1185, "X min (V)"=w1106, "X max (V)"=w1105) -> (w1126:T13)  [unwired: 1 out]
                  n558 = local read "Detector A"() -> (w1169:bool)
                  n559 = local read "Detector B"() -> (w1168:bool)
                  n560 = local read "Detector C"() -> (w1104:bool)
                  n561 = local read "Detector D"() -> (w1103:bool)
                  n562 = Open/Create/Replace File(file path (use dialog)=w1031, operation (0:open)=T11."replace or create") -> (refnum out=w1194:refnum<file>, error out=w1193:errorcluster)  [unwired: 1 in, 4 out]
                  n563 = local read "SEM parameters"() -> (w1111:T2)
                  n564 = local read "FIB parameters"() -> (w1166:T3)
                  n565 = Initialize Array(0.0 ("element"), 128 ("dimension size")) -> (w1190:dbl[])
                  n566 = local read "Detector number"() -> (w1122:u8)
                  n567 = Unbundle By Name(w1126) -> ("X resolution"=w1123:u32, "Y resolution"=w1124:u32, "AO rate"=w1125:dbl)
                  n568 = Unbundle By Name(w1111) -> ("Detector A"=w1110:string, "Detector B"=w1109:string, "Brightness A"=w1088:sgl, "Contrast A"=w1087:sgl, "Brightness B"=w1107:sgl, "Contrast B"=w1108:sgl, "Magnification"=w1086:sgl, "Pixel size"=w1085:sgl, "Working distance"=w1084:sgl, "EHT"=w1083:sgl, "Aperture"=w1082:u8, "High current mode"=w1081:u8, "Probe current"=w1080:sgl, "Beam shift X"=w1075:sgl, "Beam shift Y"=w1074:sgl, "Stig X"=w1079:sgl, "Stig Y"=w1078:sgl, "Alignment X"=w1077:sgl, "Alignment Y"=w1076:sgl)
                  n569 = local read "Z-step (nm)"() -> (w1089:dbl)
                  n570 = Bundle("Detector A"=w1169, "Detector B"=w1168, "Detector C"=w1104, "Detector D"=w1103) -> (w1167:T14)  [unwired: 1 out]
                  n571 = Write to Binary File(file (use dialog)=w1194, data=w1190, error in=w1193, 5:FALSE ("prepend array or string size? (T)")) -> (refnum out=w1189:refnum<file>, error out=w1188:errorcluster)  [unwired: 3 out]
                  n572 = local read "Notes"() -> (w1090:string)
                  n573 = local read "Detector C name"() -> (w1099:string)
                  n574 = local read "Detector D name"() -> (w1100:string)
                  n575 = local read "Notes"() -> (w1115:string)
                  n576 = flat-sequence {
                    tunnel: w1094 -> [w1234]
                    tunnel: [w1234] -> w1093
                    tunnel: w1092 -> [w1233]
                    tunnel: [w1233] -> w1091
                    frame #0 {
                      "Header done?" <- TRUE ("Header done?")
                    }
                  }
                  n577 = Get Date/Time In Seconds() -> (seconds since 1Jan1904=w1133:timestamp)
                  n578 = Bundle("Detector C name"=w1099, "Detector D name"=w1100) -> (w1102:T15)  [unwired: 1 out]
                  n579 = call "Zeiss File Header.vi"("refnum"=w1189, "Notes"=w1090, "Other detectors"=w1102, "task"=w1095, "Resolution and scan"=w1126, "AI channels"=w1167, "error in"=w1188, "SEM parameters"=w1111, "FIB parameters"=w1166) -> ("dup refnum"=w1094:refnum<file>, "error out"=w1092:errorcluster)  [unwired: 5 out]
                  n580 = Get Date/Time String(seconds (now)=w1133) -> (date string=w1121:string, time string=w1120:string)  [unwired: 2 out]
                  n581 = Concatenate Strings(w1113, w1115, w1113) -> (w1114:string)
                  n582 = local read "Detector A"() -> (w1071:bool)
                  n583 = local read "Detector C"() -> (w1070:bool)
                  n584 = local read "Detector D"() -> (w1069:bool)
                  n585 = local read "X resolution"() -> (w1067:u32)
                  n586 = local read "Y resolution"() -> (w1066:u32)
                  n587 = local read "Detector B"() -> (w1072:bool)
                  n588 = Multiply(x=w1067, y=w1066) -> (x*y=w1065:u32)
                  n589 = Build Array(w1071, w1072, w1070, w1069) -> (w1073:bool[])
                  n590 = local read "Detector A"() -> (w1035:bool)
                  n591 = local read "Detector B"() -> (w1034:bool)
                  n592 = local read "Detector C"() -> (w1033:bool)
                  n593 = local read "Detector D"() -> (w1032:bool)
                  n594 = Set File Position(offset (in bytes) (0)=i64 1024, refnum=w1093, from (0:start)=enum16{"start", "end", "current"}."start", error in=w1091) -> (refnum out=w1197:refnum<file>, error out=w1196:errorcluster)
                  n595 = Initialize Array(i16 0 ("element"), w1065) -> (w1039:i16[])
                  n596 = Initialize Array(i16 0 ("element"), 1 ("dimension size")) -> (w1036:i16[])
                  n597 = Boolean Array To Number(Boolean array=w1073) -> (number=w1068:u32)
                  n598 = local read "File path"() -> (w1132:path)
                  n599 = Get Date/Time In Seconds() -> (seconds since 1Jan1904=w1150:timestamp)
                  n600 = Get Date/Time In Seconds() -> (seconds since 1Jan1904=w1152:timestamp)
                  n601 = Get Date/Time In Seconds() -> (seconds since 1Jan1904=w1157:timestamp)
                  n602 = Select(t=w1039, s=w1035, f=w1036) -> (s? t:f=w1043:i16[])
                  n603 = Select(t=w1039, s=w1034, f=w1036) -> (s? t:f=w1042:i16[])
                  n604 = Select(t=w1039, s=w1033, f=w1036) -> (s? t:f=w1041:i16[])
                  n605 = Select(t=w1039, s=w1032, f=w1036) -> (s? t:f=w1040:i16[])
                  n606 = while {
                    tunnel: w1197 -> [w1274]
                    tunnel: [w1272] -> w1178
                    tunnel: w1196 -> [w1271]
                    tunnel: [w1267] -> w1177
                    tunnel: w1098 -> [w1264]
                    tunnel: [w1263] -> w1173
                    tunnel: [w1257] -> w1097
                    tunnel: [w1256] -> w1096
                    tunnel: w1068 -> [w1254]
                    shift-right: [w1252] -> w1063
                    shift-left: w1043 -> [w1251]
                    shift-right: [w1248] -> w1058
                    shift-left: w1042 -> [w1247]
                    shift-right: [w1245] -> w1057
                    shift-left: w1041 -> [w1244]
                    shift-right: [w1243] -> w1056
                    shift-left: w1040 -> [w1241]
                    i -> [w1240]
                    stop <- w1268 stop-if-true
                    n607 = Dequeue Element(queue=w1264) -> (queue out=w1257:refnum<queue>, element=w1253:i16[], error out=w1256:errorcluster)  [unwired: 1 in, 2 out]
                    n608 = local read "Detector A"() -> (w1237:bool)
                    n609 = local read "Detector B"() -> (w1236:bool)
                    n610 = local read "Detector C"() -> (w1238:bool)
                    n611 = local read "Detector D"() -> (w1239:bool)
                    n612 = local read "Y resolution"() -> (w1259:u32)
                    n613 = case shown="4" w1254 {
                      tunnel: w1253 -> [w1304 w1305 w1308 w1309 w1312 w1315 w1319 w1320 w1323 w1326 w1330 w1333 w1337 w1338 w1342]
                      tunnel: [w1304 _ w1307 _ w1311 _ w1318 _ w1322 _ w1329 _ w1334 _ w1346] -> w1250
                      tunnel: [_ w1305 w1306 _ _ w1314 w1317 _ _ w1325 w1327 _ _ w1340 w1343] -> w1249
                      tunnel: [_ _ _ w1309 w1310 w1313 w1316 _ _ _ _ w1331 w1335 w1339 w1344] -> w1246
                      tunnel: [_ _ _ _ _ _ _ w1320 w1321 w1324 w1328 w1332 w1336 w1341 w1345] -> w1242
                      frame 1, Default {
                      }
                      frame 2 {
                      }
                      frame 3 {
                        n614 = Decimate 1D Array(w1308) -> (w1307:i16[], w1306:i16[])
                      }
                      frame 4 {
                      }
                      frame 5 {
                        n615 = Decimate 1D Array(w1312) -> (w1311:i16[], w1310:i16[])
                      }
                      frame 6 {
                        n616 = Decimate 1D Array(w1315) -> (w1314:i16[], w1313:i16[])
                      }
                      frame 7 {
                        n617 = Decimate 1D Array(w1319) -> (w1318:i16[], w1317:i16[], w1316:i16[])
                      }
                      frame 8 {
                      }
                      frame 9 {
                        n618 = Decimate 1D Array(w1323) -> (w1322:i16[], w1321:i16[])
                      }
                      frame 10 {
                        n619 = Decimate 1D Array(w1326) -> (w1325:i16[], w1324:i16[])
                      }
                      frame 11 {
                        n620 = Decimate 1D Array(w1330) -> (w1329:i16[], w1327:i16[], w1328:i16[])
                      }
                      frame 12 {
                        n621 = Decimate 1D Array(w1333) -> (w1331:i16[], w1332:i16[])
                      }
                      frame 13 {
                        n622 = Decimate 1D Array(w1337) -> (w1334:i16[], w1335:i16[], w1336:i16[])
                      }
                      frame 14 {
                        n623 = Decimate 1D Array(w1338) -> (w1340:i16[], w1339:i16[], w1341:i16[])
                      }
                      frame 15 {
                        n624 = Decimate 1D Array(w1342) -> (w1346:i16[], w1343:i16[], w1344:i16[], w1345:i16[])
                      }
                    }
                    n625 = Increment(x=w1240) -> (x+1=w1260:i32)
                    n626 = To Long Integer(number=w1259) -> (32bit integer=w1258:i32)
                    n627 = Less Or Equal?(x=w1258, y=w1260) -> (x <= y?=w1261:bool)
                    n628 = Write to Binary File(file (use dialog)=w1274, data=w1253, error in=w1271, 5:FALSE ("prepend array or string size? (T)")) -> (refnum out=w1273:refnum<file>, error out=w1270:errorcluster)  [unwired: 3 out]
                    n629 = Unbundle By Name(w1256) -> ("status"=w1262:bool)
                    n630 = case shown="True" w1237 {
                      tunnel: [w1297 w1303] -> w1252
                      tunnel: w1251 -> [w1297 w1302]
                      tunnel: w1250 -> [_ w1301]
                      tunnel: w1240 -> [_ w1299]
                      frame False {
                      }
                      frame True {
                        n631 = Array Size(array=w1301) -> (size(s)=w1300:i32)
                        n632 = Multiply(x=w1300, y=w1299) -> (x*y=w1298:i32)
                        n633 = Replace Array Subset(array=w1302, new element=w1301, index=w1298) -> (w1303:i16[])
                      }
                    }
                    n634 = case shown="True" w1236 {
                      tunnel: [w1290 w1296] -> w1248
                      tunnel: w1247 -> [w1290 w1295]
                      tunnel: w1249 -> [_ w1294]
                      tunnel: w1240 -> [_ w1292]
                      frame False {
                      }
                      frame True {
                        n635 = Array Size(array=w1294) -> (size(s)=w1293:i32)
                        n636 = Multiply(x=w1293, y=w1292) -> (x*y=w1291:i32)
                        n637 = Replace Array Subset(array=w1295, new element=w1294, index=w1291) -> (w1296:i16[])
                      }
                    }
                    n638 = case shown="True" w1238 {
                      tunnel: [w1283 w1289] -> w1245
                      tunnel: w1244 -> [w1283 w1288]
                      tunnel: w1246 -> [_ w1287]
                      tunnel: w1240 -> [_ w1285]
                      frame False {
                      }
                      frame True {
                        n639 = Array Size(array=w1287) -> (size(s)=w1286:i32)
                        n640 = Multiply(x=w1286, y=w1285) -> (x*y=w1284:i32)
                        n641 = Replace Array Subset(array=w1288, new element=w1287, index=w1284) -> (w1289:i16[])
                      }
                    }
                    n642 = case shown="True" w1239 {
                      tunnel: [w1276 w1282] -> w1243
                      tunnel: w1241 -> [w1276 w1281]
                      tunnel: w1242 -> [_ w1280]
                      tunnel: w1240 -> [_ w1278]
                      frame False {
                      }
                      frame True {
                        n643 = Array Size(array=w1280) -> (size(s)=w1279:i32)
                        n644 = Multiply(x=w1279, y=w1278) -> (x*y=w1277:i32)
                        n645 = Replace Array Subset(array=w1281, new element=w1280, index=w1277) -> (w1282:i16[])
                      }
                    }
                    n646 = Get File Position(4:w1270, 7:w1273) -> (0:w1267:errorcluster, 2:w1263:i64, 3:w1272:refnum<file>)
                    n647 = Unbundle By Name(w1267) -> ("status"=w1269:bool)
                    n648 = local read "Save"() -> (w1266:bool)
                    n649 = local read "stop"() -> (w1255:bool)
                    n650 = Not(x=w1266) -> (.not. x?=w1265:bool)
                    n651 = Compound Arithmetic op=OR(w1269, w1262, w1265, w1261, w1255) -> (w1268:bool)
                  }
                  n652 = Format Date/Time String(time format string (%c)="Y%Y\\%Y", seconds (now)=w1150) -> (date/time string=w1151:string)  [unwired: 1 out]
                  n653 = Format Date/Time String(time format string (%c)="Y%Y\\M%m\\%Y-%m", seconds (now)=w1152) -> (date/time string=w1162:string)  [unwired: 1 out]
                  n654 = Format Date/Time String(time format string (%c)="Y%Y\\M%m\\D%d\\%Y-%m-%d", seconds (now)=w1157) -> (date/time string=w1161:string)  [unwired: 1 out]
                  n655 = Concatenate Strings(w1151, w1129) -> (w1163:string)
                  n656 = Concatenate Strings(w1162, w1129) -> (w1164:string)
                  n657 = Concatenate Strings(w1161, w1129) -> (w1165:string)
                  n658 = Build Path(base path=w1132, name or relative path=w1163) -> (appended path=w1136:path)
                  n659 = Build Path(base path=w1132, name or relative path=w1164) -> (appended path=w1154:path)
                  n660 = Build Path(base path=w1132, name or relative path=w1165) -> (appended path=w1155:path)
                  n661 = Open/Create/Replace File(file path (use dialog)=w1136, operation (0:open)=w1131) -> (refnum out=w1138:refnum<file>, error out=w1139:errorcluster)  [unwired: 1 in, 4 out]
                  n662 = Open/Create/Replace File(file path (use dialog)=w1154, operation (0:open)=w1131) -> (refnum out=w1147:refnum<file>, error out=w1146:errorcluster)  [unwired: 1 in, 4 out]
                  n663 = Open/Create/Replace File(file path (use dialog)=w1155, operation (0:open)=w1131) -> (refnum out=w1158:refnum<file>)  [unwired: 1 in, 5 out]
                  n664 = Set File Position(refnum=w1138, from (0:start)=w1130, error in=w1139) -> (refnum out=w1140:refnum<file>, error out=w1137:errorcluster)  [unwired: 1 out]
                  n665 = Set File Position(refnum=w1147, from (0:start)=w1130, error in=w1146) -> (refnum out=w1145:refnum<file>, error out=w1148:errorcluster)  [unwired: 1 out]
                  n666 = Set File Position(refnum=w1158, from (0:start)=w1130) -> (refnum out=w1159:refnum<file>)  [unwired: 1 in, 2 out]
                  n667 = local read "Y resolution"() -> (w1055:u32)
                  n668 = local read "X resolution"() -> (w1054:u32)
                  n669 = local read "Detector A"() -> (w1062:bool)
                  n670 = local read "Detector B"() -> (w1059:bool)
                  n671 = local read "Detector C"() -> (w1060:bool)
                  n672 = local read "Detector D"() -> (w1061:bool)
                  n673 = Set File Position(offset (in bytes) (0)=i64 1000, refnum=w1178, from (0:start)=enum16{"start", "end", "current"}."start", error in=w1177) -> (refnum out=w1181:refnum<file>, error out=w1176:errorcluster)
                  n674 = case shown="True" w1062 {
                    tunnel: w1063 -> [_ w1232]
                    tunnel: w1055 -> [_ w1231]
                    tunnel: w1054 -> [_ w1230]
                    tunnel: [0.0 ("Focus index") w1228] -> w1053
                    frame False {
                    }
                    frame True {
                      n675 = Reshape Array(w1232, w1231, w1230) -> (w1229:i16[][])
                      n676 = call "Focus Index.vi"("Input"=w1229) -> ("Eval area"=w1227:dbl[][], "Focus index"=w1228:sgl)  [unwired: 9 in]
                      n677 = To Word Integer(number=w1227) -> (16bit integer=→"Eval A":i16[][])
                    }
                  }
                  n678 = case shown="True" w1059 {
                    tunnel: w1058 -> [_ w1224]
                    tunnel: w1055 -> [_ w1223]
                    tunnel: w1054 -> [_ w1222]
                    tunnel: [0.0 ("Focus index") w1220] -> w1052
                    frame False {
                    }
                    frame True {
                      n679 = Reshape Array(w1224, w1223, w1222) -> (w1221:i16[][])
                      n680 = call "Focus Index.vi"("Input"=w1221) -> ("Eval area"=w1219:dbl[][], "Focus index"=w1220:sgl)  [unwired: 9 in]
                      n681 = To Word Integer(number=w1219) -> (16bit integer=→"Eval B":i16[][])
                    }
                  }
                  n682 = case shown="True" w1060 {
                    tunnel: w1057 -> [_ w1216]
                    tunnel: w1055 -> [_ w1215]
                    tunnel: w1054 -> [_ w1214]
                    tunnel: [0.0 ("Focus index") w1212] -> w1051
                    frame False {
                    }
                    frame True {
                      n683 = Reshape Array(w1216, w1215, w1214) -> (w1213:i16[][])
                      n684 = call "Focus Index.vi"("Input"=w1213) -> ("Eval area"=w1210:dbl[][], "Focus index"=w1212:sgl)  [unwired: 9 in]
                      n685 = To Word Integer(number=w1210) -> (16bit integer=→"Eval C":i16[][])
                    }
                  }
                  n686 = case shown="True" w1061 {
                    tunnel: w1056 -> [_ w1208]
                    tunnel: w1055 -> [_ w1207]
                    tunnel: w1054 -> [_ w1206]
                    tunnel: [0.0 ("Focus index") w1204] -> w1050
                    frame False {
                    }
                    frame True {
                      n687 = Reshape Array(w1208, w1207, w1206) -> (w1205:i16[][])
                      n688 = call "Focus Index.vi"("Input"=w1205) -> ("Eval area"=w1202:dbl[][], "Focus index"=w1204:sgl)  [unwired: 9 in]
                      n689 = To Word Integer(number=w1202) -> (16bit integer=→"Eval D":i16[][])
                    }
                  }
                  n690 = Write to Binary File(file (use dialog)=w1181, data=w1173, error in=w1176, 5:FALSE ("prepend array or string size? (T)")) -> (refnum out=w1180:refnum<file>, error out=w1179:errorcluster)  [unwired: 3 out]
                  n691 = Close File(refnum=w1180, error in=w1179) -> (error out=w1187:errorcluster)  [unwired: 1 out]
                  n692 = local read "Image Focus Index"() -> (w1048:T1)
                  n693 = call <vilib>:"General Error Handler.vi"("type of dialog (OK msg:1)"=w1186, "error in (no error)"=w1187) -> ()  [unwired: 14 out]
                  n694 = Bundle(cluster=w1048, "A Img Focus Index"=w1053, "B Img Focus Index"=w1052, "C Img Focus Index"=w1051, "D Img Focus Index"=w1050) -> (w1049:T1)
                  "Image Focus Index" <- w1049
                  n695 = Unbundle By Name(w1049) -> ("A Img Focus Index"=w1047:dbl, "B Img Focus Index"=w1046:dbl, "C Img Focus Index"=w1045:dbl, "D Img Focus Index"=w1044:dbl)
                  n696 = Build Array(w1122, w1123, w1124, w1125, w1088, w1087, w1107, w1108, w1086, w1085, w1084, w1083, w1082, w1081, w1080, w1075, w1074, w1079, w1078, w1077, w1076, w1089, w1047, w1046, w1045, w1044) -> (w1128:dbl[])
                  n697 = Array To Spreadsheet String(delimiter (Tab)=",", array=w1128, 3:"%#g" ("format string")) -> (spreadsheet string=w1112:string)
                  n698 = Scan String For Tokens(9:w1112) -> (1:w1101:string)  [unwired: 1 in, 7 out]
                  n699 = Build Array(w1121, w1120, w1114, w1110, w1109, w1099, w1100, w1101) -> (w1119:string[])
                  n700 = Array To Spreadsheet String(delimiter (Tab)=",", array=w1119, 3:"%s" ("format string")) -> (spreadsheet string=w1116:string)
                  n701 = Write to Text File(file (use dialog)=w1140, text=w1116, error in=w1137) -> (refnum out=w1141:refnum<file>, error out=w1142:errorcluster)  [unwired: 2 out]
                  n702 = Write to Text File(file (use dialog)=w1145, text=w1116, error in=w1148) -> (refnum out=w1144:refnum<file>, error out=w1143:errorcluster)  [unwired: 2 out]
                  n703 = Write to Text File(file (use dialog)=w1159, text=w1116) -> (refnum out=w1160:refnum<file>)  [unwired: 1 in, 3 out]
                  n704 = Close File(refnum=w1141, error in=w1142) -> ()  [unwired: 2 out]
                  n705 = Close File(refnum=w1144, error in=w1143) -> ()  [unwired: 2 out]
                  n706 = Close File(refnum=w1160) -> ()  [unwired: 1 in, 2 out]
                }
                frame True {
                  n707 = local write "Header done?"(TRUE ("Header done?")) -> ()
                  n708 = Wait on Occurrence(2:w1347) -> ()  [unwired: 2 in, 1 out]
                }
              }
            }
            frame #3 {
              n709 = local read "Display"() -> (w1349:bool)
              n710 = case shown="True" w1349 {
                frame False {
                }
                frame True {
                  w1381 = "%s, Max/Mean/Min = %#g / %#g / %#g, Focus INdex = %#5.3f" ("format string")
                  w1421 = "%s, B&C = %#u\\% & %#u\\%, Max/Mean/Min = %#g / %#g / %#g, Focus Index = %#5.3f" ("format string")
                  n711 = local read "Detector A"() -> (w1415:bool)
                  n712 = local read "Detector C"() -> (w1413:bool)
                  n713 = local read "Detector D"() -> (w1412:bool)
                  n714 = local read "Detector B"() -> (w1414:bool)
                  n715 = case shown="True" w1415 {
                    tunnel: [u8[][] [] w1548] -> w1396
                    tunnel: [_ w1551] -> w1393
                    tunnel: [_ w1550] -> w1392
                    tunnel: [_ w1549] -> w1391
                    tunnel: [_ w1553] -> w1369
                    frame False {
                    }
                    frame True {
                      n716 = local read "Det A Img"() -> (w1552:i16[][])
                      n717 = local read "Image Focus Index"() -> (w1554:T1)
                      n718 = call "16bit Image Normalization.vi"("Input image"=w1552) -> ("min"=w1549:i16, "mean"=w1550:i16, "max"=w1551:i16, "Normalized image"=w1548:u8[][])  [unwired: 6 in, 1 out]
                      n719 = Unbundle By Name(w1554) -> ("A Img Focus Index"=w1553:dbl)
                    }
                  }
                  n720 = case shown="False" w1414 {
                    tunnel: [u8[][] [] w1544] -> w1397
                    tunnel: [_ w1543] -> w1390
                    tunnel: [_ w1542] -> w1388
                    tunnel: [_ w1541] -> w1389
                    tunnel: [_ w1545] -> w1370
                    frame False {
                    }
                    frame True {
                      n721 = local read "Det B Img"() -> (w1540:i16[][])
                      n722 = local read "Image Focus Index"() -> (w1546:T1)
                      n723 = call "16bit Image Normalization.vi"("Input image"=w1540) -> ("min"=w1541:i16, "mean"=w1542:i16, "max"=w1543:i16, "Normalized image"=w1544:u8[][])  [unwired: 6 in, 1 out]
                      n724 = Unbundle By Name(w1546) -> ("B Img Focus Index"=w1545:dbl)
                    }
                  }
                  n725 = case shown="True" w1413 {
                    tunnel: [u8[][] [] w1530] -> w1395
                    tunnel: [_ w1532] -> w1385
                    tunnel: [_ w1533] -> w1386
                    tunnel: [_ w1531] -> w1384
                    tunnel: [_ w1534] -> w1368
                    frame False {
                    }
                    frame True {
                      n726 = local read "Det C Img"() -> (w1529:i16[][])
                      n727 = local read "Image Focus Index"() -> (w1535:T1)
                      n728 = call "16bit Image Normalization.vi"("Input image"=w1529) -> ("min"=w1531:i16, "mean"=w1532:i16, "max"=w1533:i16, "Normalized image"=w1530:u8[][])  [unwired: 6 in, 1 out]
                      n729 = Unbundle By Name(w1535) -> ("C Img Focus Index"=w1534:dbl)
                    }
                  }
                  n730 = case shown="True" w1412 {
                    tunnel: [u8[][] [] w1522] -> w1394
                    tunnel: [_ w1525] -> w1380
                    tunnel: [_ w1524] -> w1379
                    tunnel: [_ w1523] -> w1378
                    tunnel: [_ w1526] -> w1367
                    frame False {
                    }
                    frame True {
                      n731 = local read "Det D Img"() -> (w1521:i16[][])
                      n732 = local read "Image Focus Index"() -> (w1527:T1)
                      n733 = call "16bit Image Normalization.vi"("Input image"=w1521) -> ("min"=w1523:i16, "mean"=w1524:i16, "max"=w1525:i16, "Normalized image"=w1522:u8[][])  [unwired: 6 in, 1 out]
                      n734 = Unbundle By Name(w1527) -> ("D Img Focus Index"=w1526:dbl)
                    }
                  }
                  n735 = Build Array(w1415, w1414, w1413, w1412) -> (w1411:bool[])
                  n736 = Boolean Array To Number(Boolean array=w1411) -> (number=w1424:u32)
                  n737 = Build Array (concatenate)(w1396, w1397, w1395, w1394) -> (w1366:u8[][])
                  n738 = local read "Detector C name"() -> (w1377:string)
                  n739 = local read "Detector D name"() -> (w1382:string)
                  n740 = local read "Inverse PNG"() -> (w1436:bool)
                  n741 = Transpose 2D Array(2D array=w1366) -> (transposed array=w1453:u8[][])
                  n742 = local read "Detector A"() -> (w1358:bool)
                  n743 = local read "Detector C"() -> (w1357:bool)
                  n744 = local read "Detector D"() -> (w1354:bool)
                  n745 = local read "Eval A"() -> (w1360:i16[][])
                  n746 = local read "Eval B"() -> (w1361:i16[][])
                  n747 = local read "Eval C"() -> (w1362:i16[][])
                  n748 = local read "Eval D"() -> (w1363:i16[][])
                  n749 = local read "Detector B"() -> (w1355:bool)
                  n750 = Array Size(array=w1453) -> (size(s)=w1456:i32[])
                  n751 = local read "SEM parameters"() -> (w1416:T2)
                  n752 = Unbundle By Name(w1416) -> ("Detector A"=w1420:string, "Brightness A"=w1372:sgl, "Contrast A"=w1371:sgl, "Detector B"=w1417:string, "Brightness B"=w1418:sgl, "Contrast B"=w1419:sgl)
                  n753 = Build Array(w1358, w1355, w1357, w1354) -> (w1356:bool[])
                  n754 = case shown="True" w1436 {
                    tunnel: [u8 0 ("element") u8 255 ("element")] -> w1457
                    frame False {
                    }
                    frame True {
                    }
                  }
                  n755 = Index Array(array=w1456, index=1) -> (element=w1352:i32)
                  n756 = Boolean Array To Number(Boolean array=w1356) -> (number=w1359:u32)
                  n757 = case shown="4" w1359 {
                    tunnel: w1360 -> [w1473 _ w1475 _ w1477 _ w1479 _ w1481 _ w1483 _ w1485 _ w1487]
                    tunnel: w1361 -> [_ w1474 _ _ _ w1478 _ _ _ w1482 _ _ _ w1486 _]
                    tunnel: [w1473 w1474 w1475 w1476 w1477 w1478 w1479 w1480 w1481 w1482 w1483 w1484 w1485 w1486 w1487] -> w1353
                    tunnel: w1362 -> [_ _ _ w1476 _ _ _ _ _ _ _ w1484 _ _ _]
                    tunnel: w1363 -> [_ _ _ _ _ _ _ w1480 _ _ _ _ _ _ _]
                    frame 1, Default {
                    }
                    frame 2 {
                    }
                    frame 3 {
                    }
                    frame 4 {
                    }
                    frame 5 {
                    }
                    frame 6 {
                    }
                    frame 7 {
                    }
                    frame 8 {
                    }
                    frame 9 {
                    }
                    frame 10 {
                    }
                    frame 11 {
                    }
                    frame 12 {
                    }
                    frame 13 {
                    }
                    frame 14 {
                    }
                    frame 15 {
                    }
                  }
                  n758 = call "16bit Image Normalization.vi"("Input image"=w1353) -> ("Normalized image"=w1365:u8[][])  [unwired: 6 in, 4 out]
                  n759 = Initialize Array(w1457, 60 ("dimension size"), w1352) -> (w1454:u8[][])
                  n760 = local read "Inverse PNG"() -> (w1364:bool)
                  n761 = local read "PNG only"() -> (w1350:bool)
                  n762 = Transpose 2D Array(2D array=w1365) -> (transposed array=w1351:u8[][])
                  n763 = Format Into String(format string=w1421, w1420, w1372, w1371, w1393, w1392, w1391, w1369) -> (resulting string=w1423:string)  [unwired: 2 in, 1 out]
                  n764 = Format Into String(format string=w1421, w1417, w1418, w1419, w1390, w1388, w1389, w1370) -> (resulting string=w1422:string)  [unwired: 2 in, 1 out]
                  n765 = Format Into String(format string=w1381, w1377, w1386, w1385, w1384, w1368) -> (resulting string=w1387:string)  [unwired: 2 in, 1 out]
                  n766 = Format Into String(format string=w1381, w1382, w1380, w1379, w1378, w1367) -> (resulting string=w1383:string)  [unwired: 2 in, 1 out]
                  n767 = Unbundle By Name(w1416) -> ("Magnification"=w1376:sgl, "Pixel size"=w1375:sgl, "Working distance"=w1374:sgl, "EHT"=w1373:sgl)
                  n768 = case shown="False" w1364 {
                    tunnel: [u32[] [16777222, 65793, 131586, 197379, 263172, 328965, 394758, 460551, 526344, 592137, 657930, 723723, 789516, 855309, 921102, 986895, 1052688, 1118481, 1184274, 1250067, 1315860, 1381653, 1447446, 1513239, 1579032, 1644825, 1710618, 1776411, 1842204, 1907997, 1973790, 2039583, 2105376, 2171169, 2236962, 2302755, 2368548, 2434341, 2500134, 2565927, 2631720, 2697513, 2763306, 2829099, 2894892, 2960685, 3026478, 3092271, 3158064, 3223857, 3289650, 3355443, 3421236, 3487029, 3552822, 3618615, 3684408, 3750201, 3815994, 3881787, 3947580, 4013373, 4079166, 4144959, 4210752, 4276545, 4342338, 4408131, 4473924, 4539717, 4605510, 4671303, 4737096, 4802889, 4868682, 4934475, 5000268, 5066061, 5131854, 5197647, 5263440, 5329233, 5395026, 5460819, 5526612, 5592405, 5658198, 5723991, 5789784, 5855577, 5921370, 5987163, 6052956, 6118749, 6184542, 6250335, 6316128, 6381921, 6447714, 6513507, 6579300, 6645093, 6710886, 6776679, 6842472, 6908265, 6974058, 7039851, 7105644, 7171437, 7237230, 7303023, 7368816, 7434609, 7500402, 7566195, 7631988, 7697781, 7763574, 7829367, 7895160, 7960953, 8026746, 8092539, 8158332, 8224125, 8289918, 8355711, 8421504, 8487297, 8553090, 8618883, 8684676, 8750469, 8816262, 8882055, 8947848, 9013641, 9079434, 9145227, 9211020, 9276813, 9342606, 9408399, 9474192, 9539985, 9605778, 9671571, 9737364, 9803157, 9868950, 9934743, 10000536, 10066329, 10132122, 10197915, 10263708, 10329501, 10395294, 10461087, 10526880, 10592673, 10658466, 10724259, 10790052, 10855845, 10921638, 10987431, 11053224, 11119017, 11184810, 11250603, 11316396, 11382189, 11447982, 11513775, 11579568, 11645361, 11711154, 11776947, 11842740, 11908533, 11974326, 12040119, 12105912, 12171705, 12237498, 12303291, 12369084, 12434877, 12500670, 12566463, 12632256, 12698049, 12763842, 12829635, 12895428, 12961221, 13027014, 13092807, 13158600, 13224393, 13290186, 13355979, 13421772, 13487565, 13553358, 13619151, 13684944, 13750737, 13816530, 13882323, 13948116, 14013909, 14079702, 14145495, 14211288, 14277081, 14342874, 14408667, 14474460, 14540253, 14606046, 14671839, 14737632, 14803425, 14869218, 14935011, 15000804, 15066597, 15132390, 15198183, 15263976, 15329769, 15395562, 15461355, 15527148, 15592941, 15658734, 15724527, 15790320, 15856113, 15921906, 15987699, 16053492, 16119285, 16185078, 16250871, 16316664, 16382457, 16448250, 16514043, 16579836, 16645629, 16711422, 16448250] ("256 gray scale") u32[] [16448250, 16711422, 16645629, 16579836, 16514043, 16448250, 16382457, 16316664, 16250871, 16185078, 16119285, 16053492, 15987699, 15921906, 15856113, 15790320, 15724527, 15658734, 15592941, 15527148, 15461355, 15395562, 15329769, 15263976, 15198183, 15132390, 15066597, 15000804, 14935011, 14869218, 14803425, 14737632, 14671839, 14606046, 14540253, 14474460, 14408667, 14342874, 14277081, 14211288, 14145495, 14079702, 14013909, 13948116, 13882323, 13816530, 13750737, 13684944, 13619151, 13553358, 13487565, 13421772, 13355979, 13290186, 13224393, 13158600, 13092807, 13027014, 12961221, 12895428, 12829635, 12763842, 12698049, 12632256, 12566463, 12500670, 12434877, 12369084, 12303291, 12237498, 12171705, 12105912, 12040119, 11974326, 11908533, 11842740, 11776947, 11711154, 11645361, 11579568, 11513775, 11447982, 11382189, 11316396, 11250603, 11184810, 11119017, 11053224, 10987431, 10921638, 10855845, 10790052, 10724259, 10658466, 10592673, 10526880, 10461087, 10395294, 10329501, 10263708, 10197915, 10132122, 10066329, 10000536, 9934743, 9868950, 9803157, 9737364, 9671571, 9605778, 9539985, 9474192, 9408399, 9342606, 9276813, 9211020, 9145227, 9079434, 9013641, 8947848, 8882055, 8816262, 8750469, 8684676, 8618883, 8553090, 8487297, 8421504, 8355711, 8289918, 8224125, 8158332, 8092539, 8026746, 7960953, 7895160, 7829367, 7763574, 7697781, 7631988, 7566195, 7500402, 7434609, 7368816, 7303023, 7237230, 7171437, 7105644, 7039851, 6974058, 6908265, 6842472, 6776679, 6710886, 6645093, 6579300, 6513507, 6447714, 6381921, 6316128, 6250335, 6184542, 6118749, 6052956, 5987163, 5921370, 5855577, 5789784, 5723991, 5658198, 5592405, 5526612, 5460819, 5395026, 5329233, 5263440, 5197647, 5131854, 5066061, 5000268, 4934475, 4868682, 4802889, 4737096, 4671303, 4605510, 4539717, 4473924, 4408131, 4342338, 4276545, 4210752, 4144959, 4079166, 4013373, 3947580, 3881787, 3815994, 3750201, 3684408, 3618615, 3552822, 3487029, 3421236, 3355443, 3289650, 3223857, 3158064, 3092271, 3026478, 2960685, 2894892, 2829099, 2763306, 2697513, 2631720, 2565927, 2500134, 2434341, 2368548, 2302755, 2236962, 2171169, 2105376, 2039583, 1973790, 1907997, 1842204, 1776411, 1710618, 1644825, 1579032, 1513239, 1447446, 1381653, 1315860, 1250067, 1184274, 1118481, 1052688, 986895, 921102, 855309, 789516, 723723, 657930, 592137, 526344, 460551, 394758, 328965, 263172, 197379, 131586, 65793, 16777222] ("256 gray scale inverse")] -> w1460
                    frame False {
                    }
                    frame True {
                    }
                  }
                  n769 = case shown="True" w1350 {
                    tunnel: w1454 -> [w1469 w1472]
                    tunnel: w1453 -> [w1468 w1471]
                    tunnel: [w1467 w1470] -> w1452
                    tunnel: w1351 -> [w1466 _]
                    frame False {
                      n770 = Build Array (concatenate)(w1469, w1468, w1466) -> (w1467:u8[][])
                    }
                    frame True {
                      n771 = Build Array (concatenate)(w1472, w1471) -> (w1470:u8[][])
                    }
                  }
                  n772 = local read "File name"() -> (w1465:path)
                  n773 = case shown="13" w1424 {
                    tunnel: w1423 -> [w1488 _ w1491 _ w1493 _ w1499 _ w1502 _ w1507 _ w1512 _ w1519]
                    tunnel: w1422 -> [_ w1489 w1490 _ _ w1496 w1498 _ _ w1504 w1506 _ _ w1515 w1518]
                    tunnel: w1387 -> [_ _ _ w1492 w1494 w1495 w1497 _ _ _ _ w1509 w1511 w1514 w1517]
                    tunnel: w1383 -> [_ _ _ _ _ _ _ w1500 w1501 w1503 w1505 w1508 w1510 w1513 w1516]
                    tunnel: [w1488 w1489 w1491 w1492 w1493 w1496 w1499 w1500 w1502 w1504 w1507 w1509 w1512 w1515 w1519] -> w1401
                    tunnel: [_ _ w1490 _ w1494 w1495 w1498 _ w1501 w1503 w1506 w1508 w1511 w1514 w1518] -> w1400
                    tunnel: [_ _ _ _ _ _ w1497 _ _ _ w1505 _ w1510 w1513 w1517] -> w1399
                    tunnel: [_ _ _ _ _ _ _ _ _ _ _ _ _ _ w1516] -> w1398
                    frame 1, Default {
                    }
                    frame 2 {
                    }
                    frame 3 {
                    }
                    frame 4 {
                    }
                    frame 5 {
                    }
                    frame 6 {
                    }
                    frame 7 {
                    }
                    frame 8 {
                    }
                    frame 9 {
                    }
                    frame 10 {
                    }
                    frame 11 {
                    }
                    frame 12 {
                    }
                    frame 13 {
                    }
                    frame 14 {
                    }
                    frame 15 {
                    }
                  }
                  n774 = local read "AO rate"() -> (w1431:dbl)
                  n775 = case shown="True" w1364 {
                    tunnel: [_ "Inverse"] -> w1432
                    frame False {
                    }
                    frame True {
                    }
                  }
                  n776 = call <vilib>:"Flatten Pixmap.vi"("colors"=w1460, "8-bit pixmap"=w1452) -> ("image data"=w1447:T16)  [unwired: 4 in, 5 out]
                  n777 = Strip Path(path=w1465) -> (stripped path=w1464:path, name=w1433:string)
                  n778 = call <vilib>:"Draw Flattened Pixmap.vi"("image data"=w1447) -> ("new picture"=w1450:picture)  [unwired: 1 in, 7 out]
                  n779 = Format Into String(format string="%s\n%s\nScan Rate = %#g Hz", w1433, w1432, w1431) -> (resulting string=w1430:string)  [unwired: 2 in, 1 out]
                  n780 = call <vilib>:"Draw Text at Point.vi"("text color(black)"=u32 16448250, "text"=w1430, "origin"=cluster{"x":i16, "y":i16} {"x"=10, "y"=0}, "picture"=w1450) -> ("new picture"=w1435:picture)  [unwired: 5 in, 2 out]
                  n781 = local read "X resolution"() -> (w1437:u32)
                  n782 = local read "Y resolution"() -> (w1438:u32)
                  n783 = Search and Replace String(input string=w1433, search string=".dat", replace string=".png" ("replace string (\"\")")) -> (result string=w1461:string)  [unwired: 1 in, 7 out]
                  n784 = Build Path(base path=w1464, name or relative path=w1461) -> (appended path=w1459:path)
                  n785 = Format Into String(format string="Mag = %#g X\nPixel Size = %#g nm\n%#g x %#g pixels", w1376, w1375, w1437, w1438) -> (resulting string=w1429:string)  [unwired: 2 in, 1 out]
                  n786 = call <vilib>:"Draw Text at Point.vi"("text color(black)"=u32 16448250, "text"=w1429, "origin"=cluster{"x":i16, "y":i16} {"x"=200, "y"=0}, "picture"=w1435) -> ("new picture"=w1446:picture)  [unwired: 5 in, 2 out]
                  n787 = Format Into String(format string="WD = %#g mm\nEHT = %#g kV", w1374, w1373) -> (resulting string=w1440:string)  [unwired: 2 in, 1 out]
                  n788 = call <vilib>:"Draw Text at Point.vi"("text color(black)"=u32 16448250, "text"=w1440, "origin"=cluster{"x":i16, "y":i16} {"x"=350, "y"=0}, "picture"=w1446) -> ("new picture"=w1405:picture)  [unwired: 5 in, 2 out]
                  n789 = call <vilib>:"Draw Text at Point.vi"("text color(black)"=u32 16448250, "text"=w1401, "origin"=cluster{"x":i16, "y":i16} {"x"=10, "y"=45}, "picture"=w1405) -> ("new picture"=w1404:picture)  [unwired: 5 in, 2 out]
                  n790 = call <vilib>:"Draw Text at Point.vi"("text color(black)"=u32 16448250, "text"=w1400, "origin"=cluster{"x":i16, "y":i16} {"x"=522, "y"=45}, "picture"=w1404) -> ("new picture"=w1403:picture)  [unwired: 5 in, 2 out]
                  n791 = call <vilib>:"Draw Text at Point.vi"("text color(black)"=u32 16448250, "text"=w1399, "origin"=cluster{"x":i16, "y":i16} {"x"=1034, "y"=45}, "picture"=w1403) -> ("new picture"=w1402:picture)  [unwired: 5 in, 2 out]
                  n792 = call <vilib>:"Draw Text at Point.vi"("text color(black)"=u32 16448250, "text"=w1398, "origin"=cluster{"x":i16, "y":i16} {"x"=1546, "y"=45}, "picture"=w1402) -> ("new picture"=w1406:picture)  [unwired: 5 in, 2 out]
                  n793 = call <vilib>:"Picture to Pixmap.vi"("picture"=w1406) -> ("image data"=w1448:T16)  [unwired: 3 in, 7 out]
                  n794 = call <vilib>:"Write PNG File.vi"("image data"=w1448, "path to PNG file"=w1459) -> ()  [unwired: 1 in, 9 out]
                }
              }
            }
          }
        }
      }
      n795 = call <vilib>:"DAQmx Clear Task.vi"("task in"=w477, "error in"=w476) -> ("error out"=w486:errorcluster)  [unwired: 13 out]
      n796 = Get Queue Status(queue=w418, error in (no error)=w417) -> (queue out=w420:refnum<queue>, error out=w421:errorcluster, # elements in queue=w422:i32)  [unwired: 6 out]
      n797 = case shown="True" w339 {
        tunnel: w338 -> [_ w533]
        frame False {
        }
        frame True {
          n798 = Set Occurrence(w533) -> ()
        }
      }
      n799 = Equal To 0?(x=w422) -> (x = 0?=w423:bool)
      n800 = Merge Errors(w486, w467, w485) -> (w424:errorcluster)
      n801 = case shown="False" w460 {
        tunnel: w426 -> [w1594 _]
        tunnel: w425 -> [w1593 _]
        frame False {
          n802 = Release Queue(queue=w1594, error in (no error)=w1593) -> ()  [unwired: 4 out]
        }
        frame True {
        }
      }
      n803 = Compound Arithmetic op=OR(w423, w419) -> (w414:bool)
      n804 = call <vilib>:"General Error Handler.vi"("type of dialog (OK msg:1)"=w491, "error in (no error)"=w424) -> ()  [unwired: 14 out]
      n805 = case shown="True" w414 {
        tunnel: w420 -> [_ w596]
        tunnel: w421 -> [w593 w595]
        tunnel: [w593 w594] -> _
        frame False {
        }
        frame True {
          n806 = Release Queue(queue=w596, error in (no error)=w595) -> (error out=w594:errorcluster)  [unwired: 3 out]
        }
      }
      n807 = case shown="False" w414 {
        tunnel: w416 -> [w592 _]
        tunnel: w415 -> [w591 _]
        frame False {
          n808 = Release Queue(queue=w592, error in (no error)=w591) -> ()  [unwired: 4 out]
        }
        frame True {
        }
      }
    }
    frame #3 {
      n809 = local write "Header done?"(FALSE ("Header done?")) -> ()
      n810 = local write "stop"(TRUE ("stop")) -> ()
    }
  }
